vi "TestStandSoftware.vi"(11 "notifier":refnum<notifier>) -> ()   [LabVIEW 2025]
doc: "This is the main VI for the configuration editor.Copyright 2017 National Instruments Corporation\n\nLicensed under the Apache License, Version 2.0 (the \"License\"); you may not use this file except in compliance with the License. You may obtain a copy of the License at http://www.apache.org/licenses/LICENSE-2.0\nUnless required by applicable law or agreed to in writing, software distributed under the License is distributed on an \"AS IS\" BASIS, WITHOUT WARRANTIES OR CONDITIONS OF ANY KIND, either express or implied. See the License for the specific language governing permissions and limitations under the License."
uses:
  Configuration Tools/Controls/StateCluster.ctl
  Users/Public/Documents/Sandia National Labs/TSS Plugin/CEF.lvlibp/Repository/CEF_Repository.lvclass
  Users/Public/Documents/Sandia National Labs/TSS Plugin/CEF.lvlibp/Node/NodeRef.ctl
  Users/Public/Documents/Sandia National Labs/TSS Plugin/CEF.lvlibp/Node/CEF_Node.lvclass
  Users/Public/Documents/Sandia National Labs/TSS Plugin/CEF.lvlibp/Node/StandardEvents.ctl
  Configuration Tools/Controls/FilePaths.ctl
  Users/Public/Documents/Sandia National Labs/TSS Plugin/CEF.lvlibp/glyph manager/glyph manager.ctl
  <vilib>/Utility/config.llb/Config Data RefNum.ctl
  Configuration Tools/Controls/AddMessage.ctl
  Configuration Tools/Controls/MoveMessage.ctl
  Users/Public/Documents/Sandia National Labs/TSS Plugin/CEF.lvlibp/hierarchy repo/CEF_HierarchyRepo.lvclass
  C:/Users/Public/Documents/Sandia National Labs/TSS Plugin/CEF.lvlibp/Repository/CEF_Repository.lvclass
  Users/Public/Documents/Sandia National Labs/TSS Plugin/System.lvlibp/System/System.lvclass
  Users/Public/Documents/Sandia National Labs/TSS Plugin/CEF.lvlibp/serializable node/CEF_serializable node.lvclass
  C:/Users/Public/Documents/Sandia National Labs/TSS Plugin/CEF.lvlibp/Node/CEF_Node.lvclass
  <vilib>/National Instruments/Asynchronous TDMS Logger/_Typedefs/Multiple Files Configuration.ctl
  <vilib>/National Instruments/Asynchronous TDMS Logger/_Typedefs/Multiple Files Action.ctl
  <vilib>/National Instruments/Asynchronous TDMS Logger/_Typedefs/Old Files Configuration.ctl
  <vilib>/National Instruments/Asynchronous TDMS Logger/_Typedefs/Folder Size Limit Reached.ctl
  ce7dbd15-68e1-444f-b0a0-607e461cde1a.vi
  Control Globals.vi
  Users/Public/Documents/Sandia National Labs/TSS Plugin/CEF.lvlibp/Node/ReadChildren.vi
  Users/Public/Documents/Sandia National Labs/TSS Plugin/CEF.lvlibp/Node/ReadNodeClass.vi
  C:/Users/Public/Documents/Sandia National Labs/TSS Plugin/CEF.lvlibp/hierarchy repo/CEF_HierarchyRepo.lvclass
  C:/Users/Public/Documents/Sandia National Labs/TSS Plugin/CEF.lvlibp/serializable node/CEF_serializable node.lvclass
  Configuration Tools/Config Tool.lvlib
  Users/Public/Documents/Sandia National Labs/TSS Plugin/CEF.lvlibp
  <vilib>/Utility/config.llb/NI_LVConfig.lvlib
  <vilib>/National Instruments/Asynchronous TDMS Logger/TDMS Logger.lvclass
panel:
  in  "Record":bool
  out "Time":dbl format="%<%H:%M:%S>t"
  in  "Initialize Engines":bool
  in  "File Menu":bool
  in  "TreeView":string(tree)="NID741343233"
  in  "ExecutionView Manager":refnum<k7>(container)
  in  "SequenceFileView Manager":refnum<k7>(container)
  in  "Application Manager":refnum<k7>(container)
  in  "Close Executions Btn":refnum<k7>(container)
  in  "Close Sequence File Btn":refnum<k7>(container)
  in  "Open Sequence File Btn":refnum<k7>(container)
  in  "Run Selected Sequence Btn":refnum<k7>(container)
  in  "Entry Point 2 Btn":refnum<k7>(container)
  in  "Entry Point 1 Btn":refnum<k7>(container)
  in  "Executions ComboBox":refnum<k7>(container) caption="Executions"
  in  "Sequences ComboBox":refnum<k7>(container) caption="Sequences"
  in  "Sequence Files ComboBox":refnum<k7>(container) caption="Sequence Files"
  in  "Execution View":refnum<k7>(container)
  in  "Terminate All Btn":refnum<k7>(container)
  in  "Break/Resume Btn":refnum<k7>(container)
  in  "Terminate/Restart Btn":refnum<k7>(container)
  in  "Report Viewer":refnum<k7>(container)
  in  "TS Pane":bool
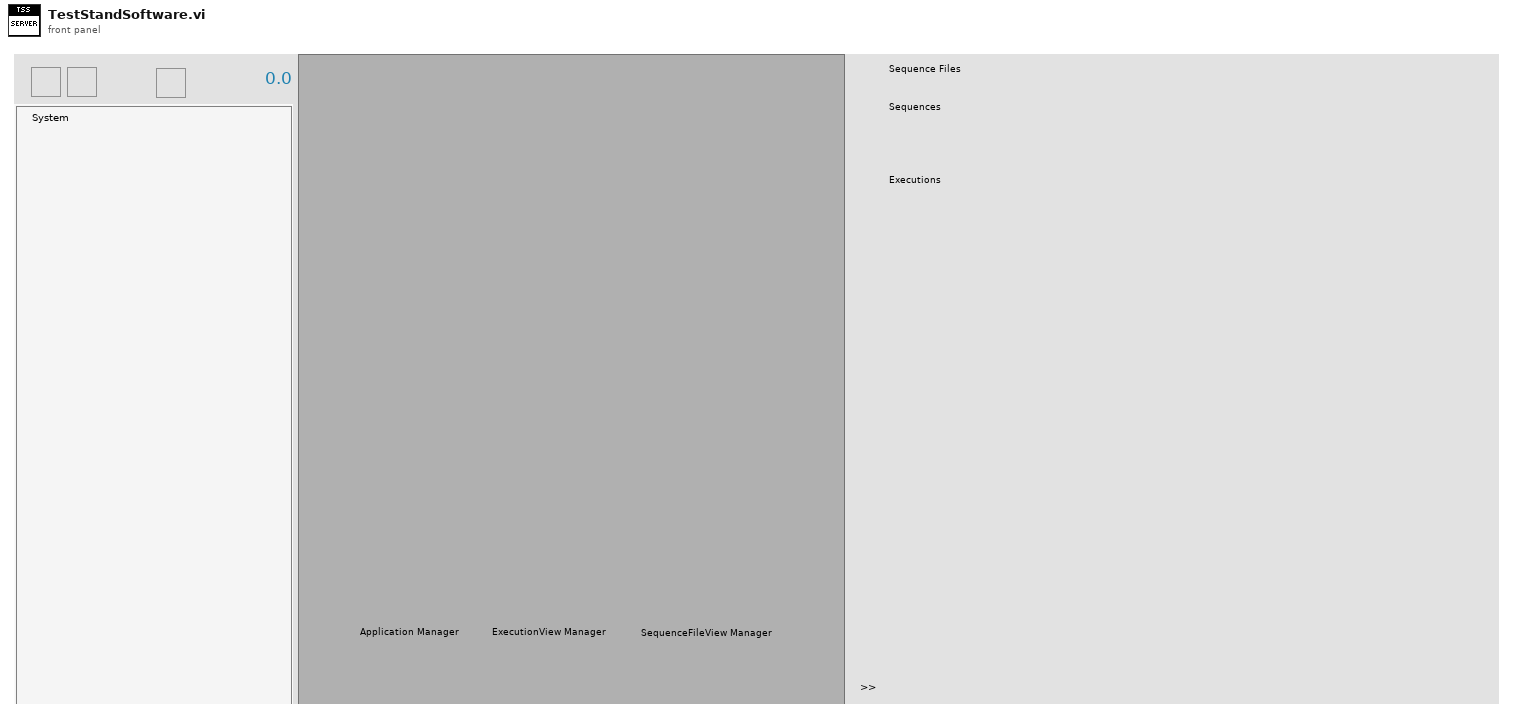
[diagram p1: front panel]
types:
  T1 = typedef "Config Tool.lvlib/StateCluster.ctl" = cluster{"repository":refnum<class "CEF_Repository.lvclass">, "root":T2, "standard events":T3, "paths":T4, "glyph manager":T5, "current path":path, "unsaved changes":bool, "menu":refnum<k9>, "Error Log":refnum<file>, "INI file ref":T6, "Record":bool, "tdms file":refnum<k34>}
  T2 = typedef "CEF.lvlibp/CEF_Node.lvclass/NodeRef.ctl" = refnum<data-value>
  T3 = typedef "CEF.lvlibp/CEF_Node.lvclass/StandardEvents.ctl" = cluster{"user event":refnum<user-event>, "node change":refnum<user-event>, "cache state":refnum<user-event>, "refresh UI":refnum<user-event>, "stop event":refnum<user-event>, "Quit App":refnum<user-event>}
  T4 = typedef "Config Tool.lvlib/FilePaths.ctl" = cluster{"Configuration":path, "Plugin":path, "Glyphs":path, "Data":path, "Error Log":path}
  T5 = typedef "CEF.lvlibp/glyph manager.ctl" = cluster{"search paths":path[], "glyph map":variant, "base glyphs":cluster{"image type":i32, "image depth":i32, "image":u8[], "mask":u8[], "colors":u32[], "Rectangle":cluster{"left":i16, "top":i16, "right":i16, "bottom":i16}}[], "desired overlays":string[]}
  T6 = typedef "NI_LVConfig.lvlib/Config Data RefNum.ctl" = refnum<k1>
  T7 = cluster{"user event":refnum<user-event>, "node change":refnum<user-event>, "cache state":refnum<user-event>, "refresh UI":refnum<user-event>, "stop event":refnum<user-event>, "Quit App":refnum<user-event>}
  T8 = typedef "Config Tool.lvlib/AddMessage.ctl" = cluster{"subNode":string, "Node ID":string}
  T9 = typedef "Config Tool.lvlib/MoveMessage.ctl" = cluster{"node ref":T2, "new parent":T2, "Index":i32}
  T10 = typedef "TDMS Logger.lvlib/TDMS Logger.lvclass/Old Files Configuration.ctl" = cluster{"Action on Max Folder Size":T11, "Max # Files in Folder":i32}
  T11 = typedef "TDMS Logger.lvlib/TDMS Logger.lvclass/Folder Size Limit Reached.ctl" = enum16{"Do Nothing", "Remove Oldest Files"}
  T12 = typedef "TDMS Logger.lvlib/TDMS Logger.lvclass/Multiple Files Configuration.ctl" = cluster{"Multiple Files Action":T13, "Max File Size (MB)":dbl, "Max Time in File (s)":dbl}
  T13 = typedef "TDMS Logger.lvlib/TDMS Logger.lvclass/Multiple Files Action.ctl" = enum16{"Seperate based on size", "Seperate based on time", "Single file"}
  T14 = cluster{"Message Name":string, "data string":string}
  T15 = typedef "LVPoint32TypeDef.ctl" = cluster{"Horizontal":i32, "Vertical":i32}
  T16 = cluster{"data name":string, "drag data":variant}[]
  T17 = cluster{"removable":bool, "movable":bool, "duplicate":bool}
  T18 = cluster{"message name":string, "data string":string}
  T19 = enum16{"Start Timer", "Read Time", "Pause", "Resume"}
  T20 = enum16{"open", "open or create", "create or replace", "create", "open (read-only)"}
  T21 = cluster{"search paths":path[], "glyph map":variant, "base glyphs":cluster{"image type":i32, "image depth":i32, "image":u8[], "mask":u8[], "colors":u32[], "Rectangle":cluster{"left":i16, "top":i16, "right":i16, "bottom":i16}}[], "desired overlays":string[]}
  T22 = cluster{"ID":string, "parent ID":string, "node type":string, "text":string, "additional text":string, "glyph":string, "depth":i32, "glyph overlay":string}[]
  T23 = cluster{"ID":string, "parent ID":string, "node type":string, "text":string, "additional text":string, "glyph":string, "depth":i32, "glyph overlay":string}
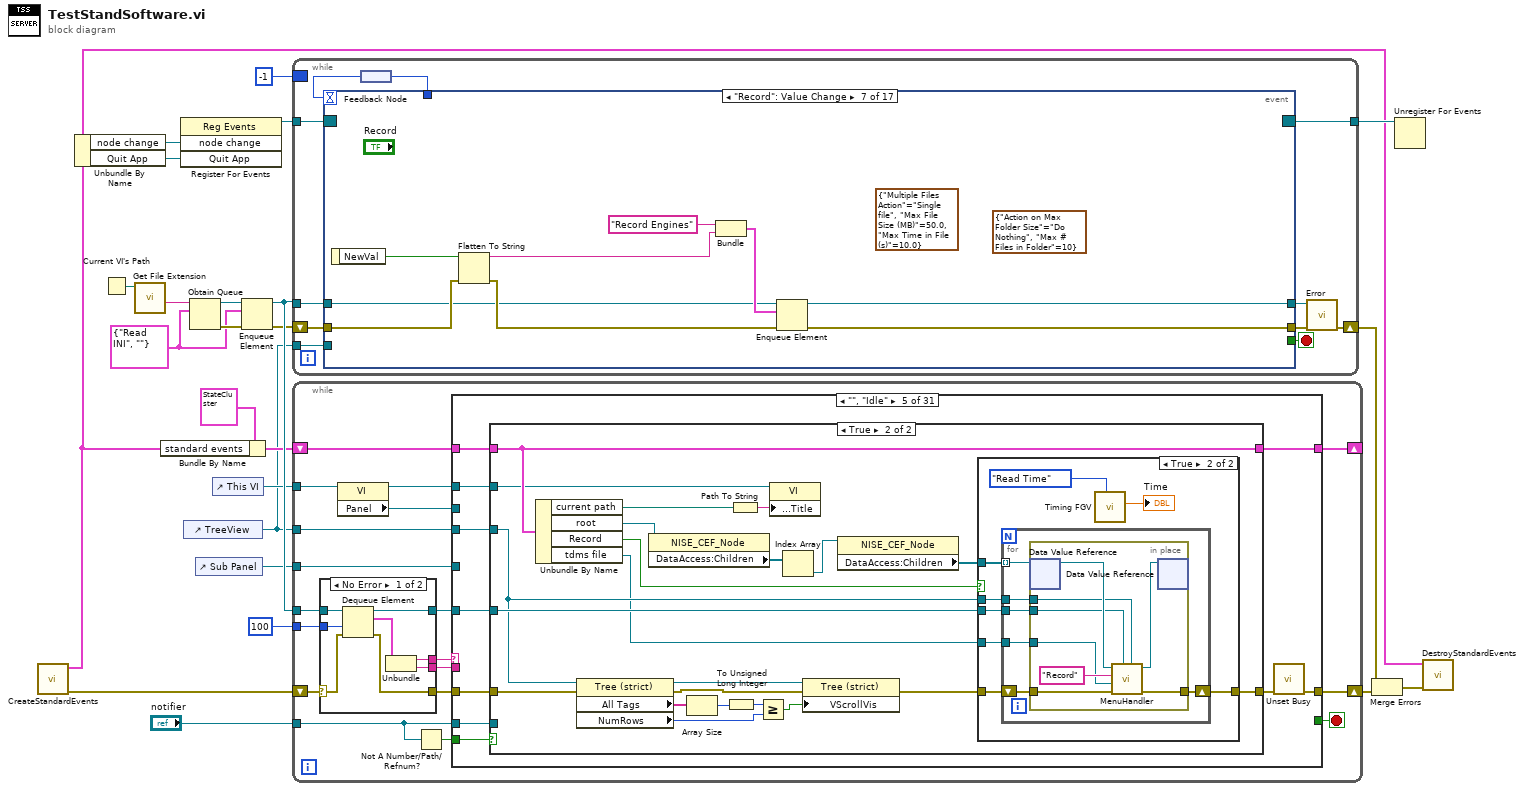
[diagram p0: block diagram]
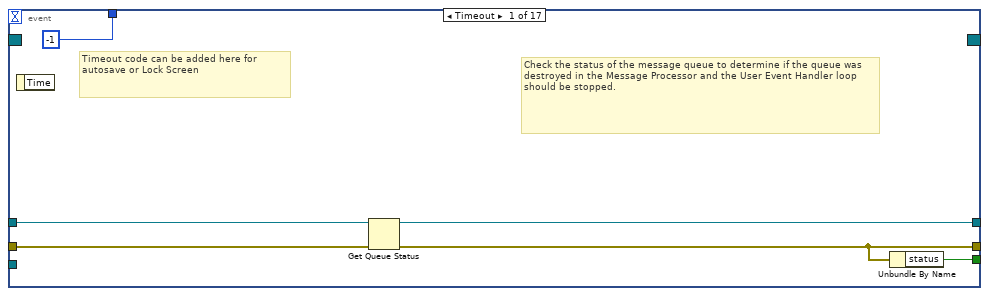
[diagram p2: hidden frame]
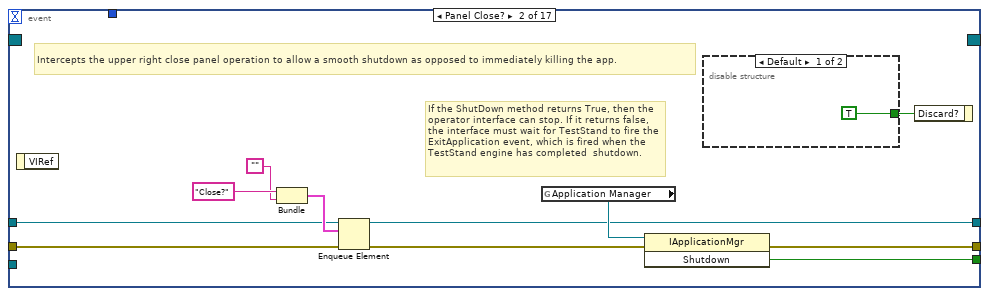
[diagram p3: hidden frame]
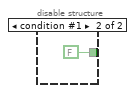
[diagram p4: hidden frame]
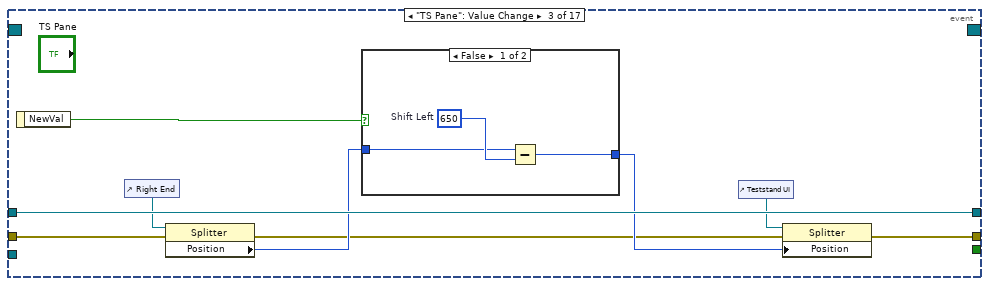
[diagram p5: hidden frame]
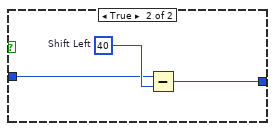
[diagram p6: hidden frame]
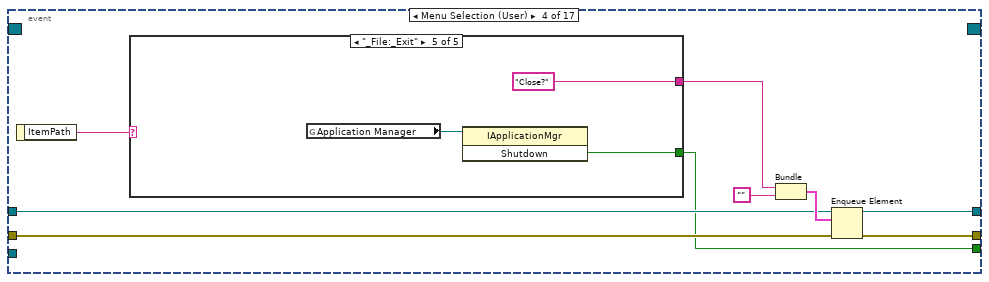
[diagram p7: hidden frame]
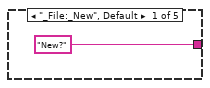
[diagram p8: hidden frame]
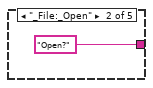
[diagram p9: hidden frame]
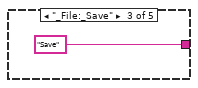
[diagram p10: hidden frame]
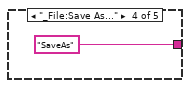
[diagram p11: hidden frame]
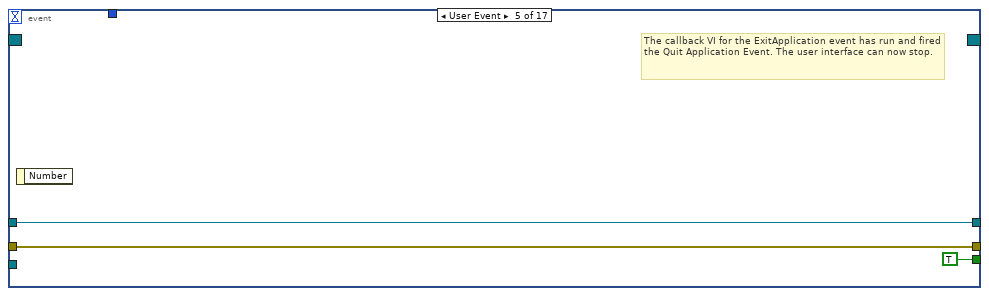
[diagram p12: hidden frame]
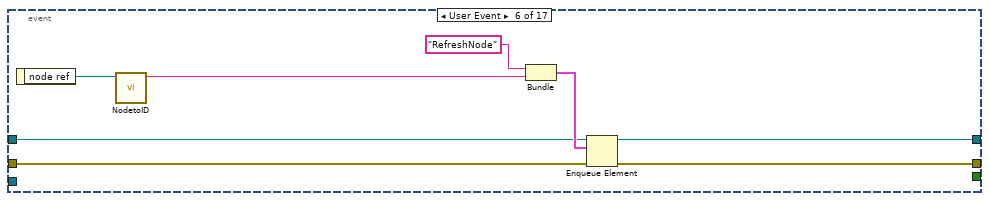
[diagram p13: hidden frame]
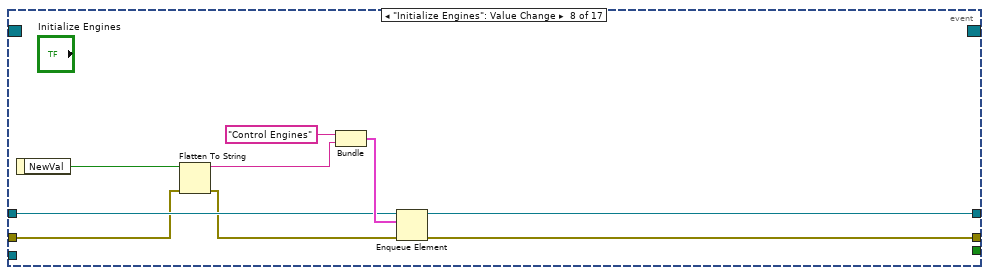
[diagram p14: hidden frame]
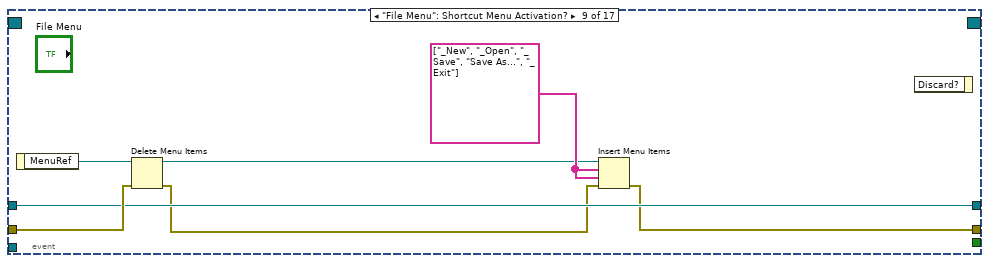
[diagram p15: hidden frame]
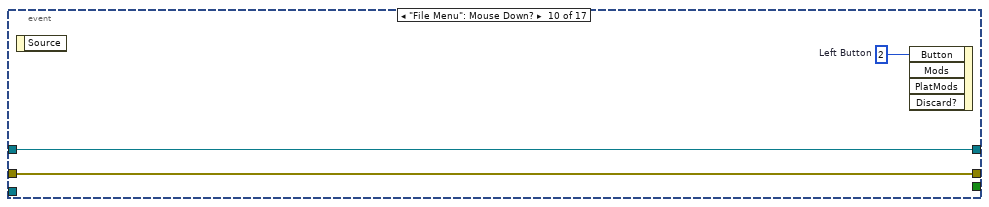
[diagram p16: hidden frame]
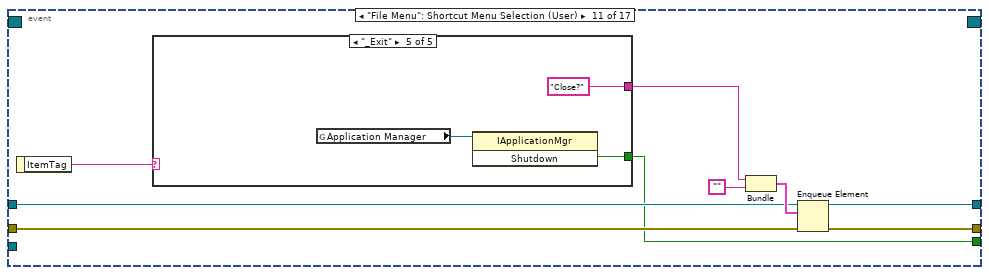
[diagram p17: hidden frame]
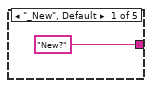
[diagram p18: hidden frame]
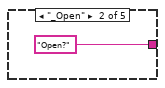
[diagram p19: hidden frame]
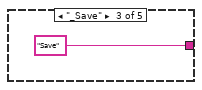
[diagram p20: hidden frame]
diagram:
  w10 = cluster{"message":string, "string":string} {"message"="Read INI", "string"=""}
  n1 = call "CreateStandardEvents.vi"() -> ("error out"=w14:errorcluster, "standard events"=w16:T7)  [unwired: 10 in]
  n2 = Unbundle By Name(w16) -> ("node change"=w15:refnum<user-event>, "Quit App"=w1:refnum<user-event>)
  n3 = Current VI's Path() -> (path=w21:path)
  n4 = call <vilib>:"Get File Extension.vi"("file"=w21) -> ("filename without extension"=w11:string)  [unwired: 6 in, 4 out]
  n5 = Bundle By Name(cluster=T1 {"repository"=refnum, "root"=refnum, "standard events"={"user event"=refnum, "node change"=refnum, "cache state"=refnum, "refresh UI"=refnum, "stop event"=refnum, "Quit App"=refnum}, "paths"={"Configuration"=path "", "Plugin"=path "", "Glyphs"=path "", "Data"=path "", "Error Log"=path ""}, "glyph manager"={"search paths"=[], "glyph map"=variant, "base glyphs"=[], "desired overlays"=[]}, "current path"=path "", "unsaved changes"=FALSE, "menu"=refnum, "Error Log"=refnum, "INI file ref"=refnum, "Record"=FALSE, "tdms file"=refnum} ("state cluster"), "standard events"=w16) -> (w4:T1)
  n6 = register-events(w15, w1) -> (reference out=w2:refnum<event-registration>)  [unwired: 2 in, 1 out]
  n7 = control-ref of="TreeView"() -> (w3:refnum<vi>)
  n8 = Obtain Queue(name (unnamed)=w11, element data type=w10) -> (queue out=w12:refnum<queue>, error out=w13:errorcluster)  [unwired: 3 in, 1 out]
  n9 = control-ref of="Sub Panel"() -> (w5:refnum<vi>)
  n10 = control-ref of="This VI"() -> (w6:refnum<vi>)
  n11 = Enqueue Element(queue=w12, element=w10, error in (no error)=w13) -> (queue out=w9:refnum<queue>, error out=w8:errorcluster)  [unwired: 1 in, 1 out]
  n12 = while "User Interface Event Handler" {
    tunnel: w9 -> [w34]
    tunnel: w3 -> [w29]
    tunnel: w2 -> [w28]
    tunnel: [w27] -> w17
    border: -1 -> [_]
    shift-right: [w31] -> w22
    shift-left: w8 -> [w35]
    stop <- w33 stop-if-true
    n13 = feedback #1() -> (w25:i32)
    n14 = event shown="[6] \"Record\": Value Change" {
      selector: w28 -> [_ _ _ _ _ _ _ _ _ _ _ _ _ _ _ _ _]
      dyn-events: [_ _ _ _ _ _ _ _ _ _ _ _ _ _ _ _ _] -> w27
      timeout: w25 -> [_ _ _ _ _ _ _ _ _ _ _ _ _ _ _ _ _]
      tunnel: [w36 w49 _ w71 TRUE ("Shutdown") _ _ _ _ _ w127 _ _ _ _ _ _] -> w33
      tunnel: [w37 w51 w62 w78 w90 w97 w101 w108 w117 w124 w128 w159 w182 w211 w239 w250 w286] -> w32
      tunnel: w35 -> [w38 w45 w57 w72 w90 w91 w103 w110 w123 w124 w129 w150 w181 w210 w237 w251 w287]
      tunnel: w34 -> [w41 w44 w64 w73 w89 w93 w102 w114 w121 w125 w131 w148 w177 w209 w236 w245 w280]
      tunnel: [w40 w43 w64 w77 w89 w92 w100 w113 w121 w125 w130 w148 w176 w209 w236 _ w279] -> w30
      tunnel: w29 -> [_ _ _ _ _ _ _ _ _ _ _ w146 _ _ _ _ _]
      tunnel: [-1 _ _ _ _ _ _ _ _ _ _ _ _ _ _ _ _] -> w26
      event Timeout {
        # "Check the status of the message queue to determine if the queue was destroyed in the Message Processor and the User Event Handler loop should be stopped."
        # "Timeout code can be added here for autosave or Lock Screen"
        n15 = event-data() -> ()  [unwired: 1 in, 1 out]
        n16 = Get Queue Status(queue=w41, error in (no error)=w38) -> (queue out=w40:refnum<queue>, error out=w37:errorcluster)  [unwired: 1 in, 6 out]
        n17 = Unbundle By Name(w37) -> ("status"=w36:bool)
      }
      event Panel Close? {
        # "If the ShutDown method returns True, then the operator interface can stop. If it returns false, the interface must wait for TestStand to fire the ExitApplication event, which is fired when the TestStand engine has completed  shutdown."
        # "Intercepts the upper right close panel operation to allow a smooth shutdown as opposed to immediately killing the app."
        n18 = event-data() -> ()  [unwired: 1 in, 1 out]
        n19 = Bundle("Close?", "") -> (w48:cluster{string, string})  [unwired: 1 in]
        n20 = Enqueue Element(queue=w44, element=w48, error in (no error)=w45) -> (queue out=w43:refnum<queue>, error out=w42:errorcluster)  [unwired: 1 in, 1 out]
        n21 = global read "Control Globals.vi" "Application Manager"() -> (w50:refnum<k7>)
        n22 = global read "Control Globals.vi" "Application Manager"() -> (w52:refnum<k7>)
        n23 = invoke class="IApplicationMgr" method="Shutdown"(reference=w50, error in=w42) -> ()  [unwired: 1 in, 3 out]
        n24 = invoke class="IApplicationMgr" method="Shutdown"(reference=w52) -> (error out=w51:errorcluster, "Shutdown"=w49:bool)  [unwired: 2 in, 1 out]
        n25 = disable-structure shown="Default" {
          disable-tunnel: [TRUE FALSE] -> w53
          frame condition #0 (active) {
          }
          frame condition #1 {
          }
        }
        n26 = event-data("Discard?"=w53) -> ()  [unwired: 1 in, 1 out]
      }
      event "TS Pane": Value Change {
        n27 = event-data() -> ("NewVal"=w60:bool)  [unwired: 1 in]
        n28 = control-ref of="Right End"() -> (w61:refnum<vi>)
        n29 = property class="Splitter"(reference=w61, error in=w57) -> (error out=w56:errorcluster, "Position"=w59:i32)  [unwired: 1 out]
        n30 = case shown="False" w60 {
          tunnel: w59 -> [w66 w69]
          tunnel: [w65 w68] -> w58
          frame False {
            w67 = 650  # Shift Left
            n31 = Subtract(x=w66, y=w67) -> (x-y=w65:i32)
          }
          frame True {
            w70 = 40  # Shift Left
            n32 = Subtract(x=w69, y=w70) -> (x-y=w68:i32)
          }
        }
        n33 = control-ref of="Teststand UI"() -> (w63:refnum<vi>)
        n34 = property class="Splitter"(reference=w63, error in=w56, "Position"=w58) -> (error out=w62:errorcluster)  [unwired: 1 out]
      }
      event Menu Selection (User) {
        n35 = event-data() -> ("ItemPath"=w79:string)  [unwired: 1 in]
        n36 = case shown="\"_File:_Exit\"" w79 {
          tunnel: ["New?" ("Message Name") "Open?" ("Message Name") "Save" ("Message Name") "SaveAs" ("Message Name") "Close?" ("Message Name")] -> w75
          tunnel: [_ _ _ _ w84] -> w71
          frame "_File:_New", Default {
          }
          frame "_File:_Open" {
          }
          frame "_File:_Save" {
          }
          frame "_File:Save As..." {
          }
          frame "_File:_Exit" {
            n37 = global read "Control Globals.vi" "Application Manager"() -> (w85:refnum<k7>)
            n38 = global read "Control Globals.vi" "Application Manager"() -> (w86:refnum<k7>)
            n39 = invoke class="IApplicationMgr" method="Shutdown"(reference=w85) -> ("Shutdown"=w84:bool)  [unwired: 2 in, 2 out]
            n40 = invoke class="IApplicationMgr" method="Shutdown"(reference=w86) -> ()  [unwired: 2 in, 3 out]
          }
        }
        n41 = Bundle("Message Name"=w75, "") -> (w74:cluster{"Message Name":string, string})  [unwired: 1 in]
        n42 = Enqueue Element(queue=w73, element=w74, error in (no error)=w72) -> (queue out=w77:refnum<queue>, error out=w78:errorcluster)  [unwired: 1 in, 1 out]
      }
      event User Event {
        # "The callback VI for the ExitApplication event has run and fired the Quit Application Event. The user interface can now stop."
        n43 = event-data() -> ()  [unwired: 1 in, 1 out]
      }
      event User Event {
        n44 = event-data() -> ("node ref"=w98:refnum<data-value>)  [unwired: 1 in]
        n45 = call "NodetoID.vi"("node ref"=w98) -> ("ID"=w94:string)  [unwired: 9 in, 1 out]
        n46 = Bundle("message name"="RefreshNode", "ID"=w94) -> (w95:cluster{"message name":string, "ID":string})  [unwired: 1 in]
        n47 = Enqueue Element(queue=w93, element=w95, error in (no error)=w91) -> (queue out=w92:refnum<queue>, error out=w97:errorcluster)  [unwired: 1 in, 1 out]
      }
      event "Record": Value Change {
        (unwired) T10 {"Action on Max Folder Size"=enum."Do Nothing", "Max # Files in Folder"=10} ("Old Files Configuration")
        (unwired) T12 {"Multiple Files Action"=enum."Single file", "Max File Size (MB)"=50.0, "Max Time in File (s)"=10.0} ("Multiple Files Configuration")
        n48 = event-data() -> ("NewVal"=w99:bool)  [unwired: 1 in]
        n49 = Flatten To String(anything=w99, error in (no error)=w103) -> (data string=w105:string, error out=w104:errorcluster)  [unwired: 2 in, 1 out]
        n50 = Bundle("Message Name"="Record Engines", "data string"=w105) -> (w107:T14)  [unwired: 1 in]
        n51 = Enqueue Element(queue=w102, element=w107, error in (no error)=w104) -> (queue out=w100:refnum<queue>, error out=w101:errorcluster)  [unwired: 1 in, 1 out]
      }
      event "Initialize Engines": Value Change {
        n52 = event-data() -> ("NewVal"=w112:bool)  [unwired: 1 in]
        n53 = Flatten To String(anything=w112, error in (no error)=w110) -> (data string=w111:string, error out=w109:errorcluster)  [unwired: 2 in, 1 out]
        n54 = Bundle("Message Name"="Control Engines", "data string"=w111) -> (w116:T14)  [unwired: 1 in]
        n55 = Enqueue Element(queue=w114, element=w116, error in (no error)=w109) -> (queue out=w113:refnum<queue>, error out=w108:errorcluster)  [unwired: 1 in, 1 out]
      }
      event "File Menu": Shortcut Menu Activation? {
        w120 = string[] ["_New", "_Open", "_Save", "Save As...", "_Exit"] ("item names")
        n56 = event-data() -> ("MenuRef"=w122:refnum<k9>)  [unwired: 1 in]
        n57 = Delete Menu Items(6:w123, 9:w122) -> (0:w118:errorcluster, 3:w119:refnum<k9>)  [unwired: 2 in]
        n58 = Insert Menu Items(6:w118, 7:w120, 8:w120, 9:w119) -> (0:w117:errorcluster)  [unwired: 2 in, 2 out]
        n59 = event-data() -> ()  [unwired: 2 in, 1 out]
      }
      event "File Menu": Mouse Down? {
        w126 = u16 2  # Left Button
        n60 = event-data() -> ()  [unwired: 1 in, 1 out]
        n61 = event-data("Button"=w126) -> ()  [unwired: 4 in, 1 out]
      }
      event "File Menu": Shortcut Menu Selection (User) {
        n62 = event-data() -> ("ItemTag"=w135:string)  [unwired: 1 in]
        n63 = case shown="\"_Exit\"" w135 {
          tunnel: ["New?" ("Message Name") "Open?" ("Message Name") "Save" ("Message Name") "SaveAs" ("Message Name") "Close?" ("Message Name")] -> w133
          tunnel: [_ _ _ _ w141] -> w127
          frame "_New", Default {
          }
          frame "_Open" {
          }
          frame "_Save" {
          }
          frame "Save As..." {
          }
          frame "_Exit" {
            n64 = global read "Control Globals.vi" "Application Manager"() -> (w142:refnum<k7>)
            n65 = global read "Control Globals.vi" "Application Manager"() -> (w143:refnum<k7>)
            n66 = invoke class="IApplicationMgr" method="Shutdown"(reference=w142) -> ("Shutdown"=w141:bool)  [unwired: 2 in, 2 out]
            n67 = invoke class="IApplicationMgr" method="Shutdown"(reference=w143) -> ()  [unwired: 2 in, 3 out]
          }
        }
        n68 = Bundle("Message Name"=w133, "") -> (w132:cluster{"Message Name":string, string})  [unwired: 1 in]
        n69 = Enqueue Element(queue=w131, element=w132, error in (no error)=w129) -> (queue out=w130:refnum<queue>, error out=w128:errorcluster)  [unwired: 1 in, 1 out]
      }
      event "TreeView": Shortcut Menu Activation? {
        n70 = event-data() -> ("MenuRef"=w149:refnum<k9>, "CtlRef"=w162:refnum<vi>, "Coords"=w161:T15)  [unwired: 1 in]
        n71 = invoke class="Tree (strict)" method="Point To Row Column"(reference=w162, "Point"=w161) -> ("Tag"=w160:string)  [unwired: 6 in, 7 out]
        n72 = property class="Tree (strict)"(reference=w146, error in=w150) -> (error out=w147:errorcluster, "Allow Editing Cells"=w145:bool)  [unwired: 1 out]
        n73 = call "IDtoNode.vi"("error in"=w147, "ID"=w160) -> ("error out"=w155:errorcluster, "invalid Id"=w153:bool, "node ref"=w158:refnum<data-value>)  [unwired: 7 in]
        n74 = Not(x=w153) -> (.not. x?=w144:bool)
        n75 = And(x=w144, y=w145) -> (x .and. y?=w152:bool)
        n76 = case shown="False" w152 {
          tunnel: w158 -> [_ w170]
          tunnel: w149 -> [_ w169]
          tunnel: [_ w168] -> w157
          tunnel: [_ w167] -> w156
          tunnel: w155 -> [w164 w166]
          tunnel: [w164 w166] -> w154
          tunnel: [TRUE ("Discard?") FALSE ("Discard?")] -> w151
          frame False {
          }
          frame True {
            n77 = in-place {
              in-place-border: w169 -> [w173]
              in-place-border: [w171] -> w168
              n78 = in-place-dvr #2(w170) -> (w175:refnum<class "CEF_Node.lvclass">, w172:errorcluster)
              n79 = call-dynamic "ShortcutMenu.vi"("error in"=w172, "menu ref in"=w173, "CEF_Node in"=w175) -> ("error out"=w171:errorcluster, "CEF_Node out"=w174:refnum<class "CEF_Node.lvclass">)  [unwired: 6 in, 1 out]
              n80 = in-place-dvr #2(w174) -> (w167:errorcluster)  [unwired: 1 out]
            }
          }
        }
        n81 = Merge Errors(w156, w157, w154) -> (w159:errorcluster)
        n82 = event-data("Discard?"=w151) -> ()  [unwired: 1 in, 1 out]
      }
      event "TreeView": Shortcut Menu Selection (User) {
        n83 = event-data() -> ("ItemPath"=w184:string, "CtlRef"=w187:refnum<vi>, "Coords"=w188:T15)  [unwired: 1 in]
        n84 = invoke class="Tree (strict)" method="Point To Row Column"(reference=w187, "Point"=w188) -> ("Tag"=w183:string)  [unwired: 6 in, 7 out]
        n85 = Match Pattern(string=w184, regular expression=":") -> (before substring=w186:string, after substring=w185:string)  [unwired: 1 in, 2 out]
        n86 = case shown="Default" w186 {
          selector: w186 -> [w192 _ _ _ _ _]
          tunnel: w185 -> [_ _ _ w202 _ _]
          tunnel: w183 -> [w193 w195 w197 w203 w205 w208]
          tunnel: ["CustomMenuAction" ("Message Name") "RemoveNode" ("Message Name") "Duplicate" ("Message Name") "AddNode" ("Message Name") "Import Engine" ("Message Name") "Export Engine" ("Message Name")] -> w179
          tunnel: [w190 w195 w197 w199 w205 w208] -> w180
          frame Default {
            # "Right click menu"
            n87 = Concatenate Strings(w192, ":" ("string"), w193) -> (w190:string)
          }
          frame "Remove" {
          }
          frame "Duplicate" {
          }
          frame "Add" {
            n88 = Bundle By Name(cluster=T8 {"subNode"="", "Node ID"=""} ("input cluster"), "subNode"=w202, "Node ID"=w203) -> (w200:T8)
            n89 = Flatten To String(anything=w200) -> (data string=w199:string)  [unwired: 3 in, 2 out]
          }
          frame "Import" {
          }
          frame "Export" {
          }
        }
        n90 = Bundle("Message Name"=w179, "Tag"=w180) -> (w178:cluster{"Message Name":string, "Tag":string})  [unwired: 1 in]
        n91 = Enqueue Element(queue=w177, element=w178, error in (no error)=w181) -> (queue out=w176:refnum<queue>, error out=w182:errorcluster)  [unwired: 1 in, 1 out]
      }
      event "TreeView": Drag Starting? {
        n92 = event-data() -> ("Data"=w218:T16, "CtlRef"=w220:refnum<vi>, "Coords"=w219:T15)  [unwired: 1 in]
        n93 = invoke class="Tree (strict)" method="Point To Row Column"(reference=w220, "Point"=w219) -> ("Tag"=w217:string)  [unwired: 6 in, 7 out]
        n94 = call "IDtoNode.vi"("error in"=w210, "ID"=w217) -> ("error out"=w212:errorcluster, "invalid Id"=w216:bool, "node ref"=w215:refnum<data-value>)  [unwired: 7 in]
        n95 = case shown="True" w216 {
          tunnel: w215 -> [w228 _]
          tunnel: [w225 TRUE ("Removable")] -> w213
          tunnel: w212 -> [w224 w234]
          tunnel: [w221 w234] -> w211
          frame False {
            n96 = in-place {
              in-place-border: [w231] -> w227
              in-place-border: w224 -> [w230]
              in-place-border: [w229] -> w223
              n97 = in-place-dvr #3(w228) -> (w233:refnum<class "CEF_Node.lvclass">)  [unwired: 1 out]
              n98 = call-dynamic "EditOptions.vi"("error in"=w230, "CEF_Node in"=w233) -> ("error out"=w229:errorcluster, "edit options"=w231:T17, "CEF_Node out"=w232:refnum<class "CEF_Node.lvclass">)  [unwired: 6 in, 1 out]
              n99 = in-place-dvr #3(w232) -> (w222:errorcluster)  [unwired: 1 out]
            }
            n100 = Unbundle By Name(w227) -> ("movable"=w226:bool)
            n101 = Merge Errors(w222, w223) -> (w221:errorcluster)
            n102 = Not(x=w226) -> (.not. x?=w225:bool)
          }
          frame True {
          }
        }
        n103 = event-data("Data"=w218, "Drag Mode"=enum32{"copy or move", "copy only", "move only"}."move only", "Discard?"=w213) -> ()  [unwired: 1 in, 1 out]
      }
      event "TreeView": event type 3.0.xa000003a {
        n104 = event-data() -> ("CtlRef"=w244:refnum<vi>, "Coords"=w241:T15)  [unwired: 1 in]
        n105 = invoke class="Tree (strict)" method="Point To Row Column"(reference=w244, "Point"=w241) -> (reference out=w243:refnum<vi>, "Tag"=w242:string)  [unwired: 6 in, 6 out]
        n106 = call "ValidDragDrop.vi"("error in"=w237, "Reorder"=TRUE, "drag over"=w242, "Tree Ref in"=w243) -> ("Error Out"=w239:errorcluster, "Accepted"=w240:bool)  [unwired: 6 out]
        n107 = event-data("Accepted?"=w240) -> ()  [unwired: 1 in, 1 out]
      }
      event "TreeView": Drop {
        n108 = event-data() -> ("CtlRef"=w262:refnum<vi>, "Coords"=w261:T15)  [unwired: 1 in]
        n109 = invoke class="Tree (strict)" method="Point To Row Column"(reference=w262, "Point"=w261) -> (reference out=w260:refnum<vi>, "Tag"=w257:string)  [unwired: 6 in, 6 out]
        n110 = call "ValidDragDrop.vi"("error in"=w251, "Reorder"=TRUE, "drag over"=w257, "Tree Ref in"=w260) -> ("Error Out"=w249:errorcluster, "Accepted"=w255:bool, "Drag"=w259:string, "Tree Ref out"=w264:refnum<vi>, "Moved Node"=w253:refnum<data-value>, "Position"=w252:i32, "Parent Node"=w254:refnum<data-value>, "Parent"=w256:string)
        n111 = case shown="True" w255 {
          tunnel: w259 -> [_ w276]
          tunnel: w264 -> [_ w278]
          tunnel: [_ TRUE] -> w263
          tunnel: w256 -> [_ w275]
          tunnel: w253 -> [_ w274]
          tunnel: w254 -> [_ w273]
          tunnel: w252 -> [_ w272]
          tunnel: ["Idle" ("message name") "Move" ("message name")] -> w248
          tunnel: [_ w267] -> w247
          frame False {
          }
          frame True {
            n112 = invoke class="Tree (strict)" method="Edit Tree Items.Move Item"(reference=w278, "tag"=w276, "New Parent"=w275, "New Position"=0, "Carry Children"=FALSE ("Carry Children?")) -> ()  [unwired: 2 in, 7 out]
            n113 = Bundle By Name(cluster=T9 {"node ref"=refnum, "new parent"=refnum, "Index"=0}, "Index"=w272, "node ref"=w274, "new parent"=w273) -> (w269:T9)
            n114 = Flatten To String(anything=w269) -> (data string=w267:string)  [unwired: 3 in, 2 out]
          }
        }
        n115 = Bundle("message name"=w248, "data string"=w247) -> (w246:T18)  [unwired: 1 in]
        n116 = event-data("Accepted?"=w263) -> ()  [unwired: 1 in, 1 out]
        n117 = Enqueue Element(queue=w245, element=w246, error in (no error)=w249) -> (error out=w250:errorcluster)  [unwired: 1 in, 2 out]
      }
      event "TreeView": Value Change {
        # "Don't remove"
        n118 = event-data() -> ("NewVal"=w282:string)  [unwired: 1 in]
        n119 = call "Stall Data Flow.vim"("value in"=w287, "milliseconds to wait"=u32 100) -> ("value out"=w285:errorcluster)  [unwired: 1 out]
        n120 = Bundle("Message Name"="ActivateNode", "NewVal"=w282) -> (w281:cluster{"Message Name":string, "NewVal":string})  [unwired: 1 in]
        n121 = Enqueue Element(queue=w280, element=w281, error in (no error)=w285) -> (queue out=w279:refnum<queue>, error out=w286:errorcluster)  [unwired: 1 in, 1 out]
      }
    }
    n122 = feedback-in #1(w26) -> ()
    n123 = call "Error.vi"("error in (no error)"=w32, "main queue"=w30) -> ("error out"=w31:errorcluster)  [unwired: 9 in]
  }
  n124 = while "Message Processor" {
    shift-right: [w304] -> _
    shift-left: w4 -> [w305]
    tunnel: w9 -> [w300]
    shift-right: [w291] -> w24
    shift-left: w14 -> [w296]
    tunnel: "notifier" -> [w302]
    tunnel: 100 ("timeout (1 ms)") -> [w298]
    tunnel: w6 -> [w290]
    tunnel: w3 -> [w293]
    tunnel: w5 -> [w292]
    stop <- w297 stop-if-true
    n125 = case shown="No Error" w296 {
      selector: w296 -> [w309 w316]
      tunnel: [w313 _] -> w301
      tunnel: w300 -> [w312 w317]
      tunnel: [w311 w317] -> w299
      tunnel: w298 -> [w310 _]
      tunnel: [w307 "Error" ("message")] -> w295
      tunnel: [w306 w315] -> w294
      frame No Error {
        n126 = Dequeue Element(queue=w312, timeout in ms (-1)=w310, error in (no error)=w309) -> (queue out=w311:refnum<queue>, element=w308:cluster{"message":string, "string":string}, error out=w313:errorcluster)  [unwired: 1 out]
        n127 = Unbundle(w308) -> ("message"=w307:string, "string"=w306:string)
      }
      frame Error {
        n128 = Flatten To String(anything=w316) -> (data string=w315:string)  [unwired: 3 in, 2 out]
      }
    }
    n129 = property class="VI"(reference=w290) -> (reference out=w289:refnum<vi>, "Panel"=w288:refnum<vi>)  [unwired: 1 in, 1 out]
    n130 = Not A Number/Path/Refnum?(number/path/refnum=w302) -> (NaN/Path/Refnum?=w303:bool)
    n131 = case shown="\"\", \"Idle\"" w295 {
      selector: w295 -> [_ _ _ _ _ _ w573 _ _ _ _ w638 _ _ _ _ _ _ _ _ _ _ _ _ _ _ _ _ _ _ _]
      tunnel: w294 -> [_ _ _ _ _ w505 _ _ _ _ _ _ w662 _ _ _ _ w844 w856 w891 w953 w969 w1003 w1022 w1067 w1083 _ w1107 w1138 w1207 w1245]
      tunnel: w301 -> [w319 w326 w356 w419 w443 w506 w577 w584 w598 w615 w628 w640 w670 w698 w766 w803 w823 w845 w855 w885 w962 w973 w1000 w1020 w1064 w1082 w1097 w1108 w1143 w1208 w1246]
      tunnel: [w319 w330 w352 w417 w436 w508 w570 w578 w599 w606 w628 w642 w660 w703 w769 w806 w823 w830 w865 w892 w948 w966 w987 w1025 w1059 w1085 w1097 w1102 w1146 w1196 w1242] -> w291
      tunnel: [w318 w341 w351 w428 w439 w507 w571 w594 w604 w624 w627 w631 w676 w718 w773 w805 w822 w853 w860 w890 w963 w967 w1005 w1029 w1062 w1087 w1096 w1100 w1147 w1214 w1240] -> w304
      tunnel: w305 -> [w318 w339 w351 w412 w440 w507 w571 w594 w604 w624 w627 w631 w675 w719 w774 w808 w822 w852 w861 w890 w960 w965 w1006 w1029 w1061 w1084 w1096 w1101 w1148 w1214 w1241]
      tunnel: w299 -> [_ w329 w359 w424 w438 w498 _ w587 w596 w614 _ w635 w671 w701 _ _ _ w826 _ w889 _ _ _ w1026 w1051 w1077 _ _ w1150 w1199 w1239]
      tunnel: w302 -> [_ w336 w357 w414 w445 w496 _ _ _ _ _ _ w672 _ _ _ _ _ _ w883 _ _ w991 _ _ w1069 _ _ _ w1209 _]
      tunnel: w303 -> [_ w334 w358 w413 w444 w495 _ _ _ _ _ _ w663 w699 _ _ _ _ _ _ _ _ w992 _ _ _ _ _ _ w1197 _]
      tunnel: [_ _ _ _ _ _ _ _ _ TRUE ("Exit") _ _ _ _ _ _ _ _ _ _ _ _ _ _ _ _ _ _ _ _ _] -> w297
      tunnel: w289 -> [_ _ w363 w421 w441 _ w568 _ _ w605 _ _ _ _ _ _ _ _ _ _ _ _ w993 _ _ _ _ _ _ _ _]
      tunnel: w293 -> [_ w323 _ w408 w442 _ _ _ _ _ _ _ _ _ _ _ _ w824 w854 w886 w946 w964 w996 _ _ w1073 _ _ _ w1210 w1238]
      tunnel: w292 -> [_ _ _ _ _ _ _ _ _ w620 _ _ _ _ _ _ _ _ _ _ _ _ w995 w1019 _ _ _ _ _ _ _]
      tunnel: w288 -> [_ _ _ _ _ _ _ w592 _ w619 _ _ _ _ _ _ _ _ _ _ _ _ _ w1018 _ _ _ _ _ _ _]
      frame "------------Generic Operations------------" {
        # "Dummy case to add a seperation in the Case Structure menu"
      }
      frame "Read INI" {
        w327 = "Test Config.ini"
        n132 = Bundle("Initialize", "") -> (w332:cluster{string, string})  [unwired: 1 in]
        n133 = Enqueue Element(queue=w329, element=w332, error in (no error)=w326) -> (error out=w325:errorcluster)  [unwired: 1 in, 2 out]
        n134 = case shown="False" w334 {
          tunnel: w336 -> [w348 _]
          tunnel: w325 -> [w345 w349]
          tunnel: [w344 w349] -> w322
          tunnel: w327 -> [w343 _]
          frame False {
            n135 = Bundle("notification"="Read INI", w343) -> (w346:cluster{"notification":string, string})  [unwired: 1 in]
            n136 = Send Notification(notification=w346, notifier=w348, error in (no error)=w345) -> (error out=w344:errorcluster)  [unwired: 1 out]
          }
          frame True {
          }
        }
        n137 = invoke class="Tree (strict)" method="Edit Tree Items.Delete"(reference=w323, "Delete Children"=TRUE ("Delete Children?")) -> (reference out=w321:refnum<vi>)  [unwired: 3 in, 4 out]
        n138 = call <vilib>:"Application Directory.vi"() -> ("Application Directory"=w338:path)
        n139 = Build Path(base path=w338, name or relative path=w327) -> (appended path=w342:path)
        n140 = invoke class="Tree (strict)" method="Custom Item Symbols.Revert Symbols"(reference=w321, error in=w322) -> (error out=w320:errorcluster)  [unwired: 1 in, 2 out]
        n141 = call "Read INI File.vi"("INI File"=w342) -> ("File paths"=w337:T4, "INI refnum"=w340:T6)  [unwired: 8 in, 1 out]
        n142 = Unbundle By Name(w337) -> ("Error Log"=w335:path)
        n143 = call "Log Error.vi"("Error In"=w320, "Log Path"=w335) -> ("Error Out"=w330:errorcluster, "Log refnum out"=w328:refnum<file>)  [unwired: 8 in]
        n144 = Bundle By Name(cluster=w339, "INI file ref"=w340, "paths"=w337, "Error Log"=w328) -> (w341:T1)
      }
      frame "Initialize" {
        # "Note: LabVIEW Global Variables are safe to use here because they are only written to at the start of the application and clearing them when finalizing shutdown. \n \nNote: You can right click a global and select Find » Global References to view all of the locations where a variable is accessed."
        n145 = case shown="False" w358 {
          tunnel: w357 -> [w369 _]
          tunnel: w356 -> [w366 w370]
          tunnel: [w365 w370] -> w355
          frame False {
            n146 = Bundle("notification"="Initialize", "") -> (w367:cluster{"notification":string, string})  [unwired: 1 in]
            n147 = Send Notification(notification=w367, notifier=w369, error in (no error)=w366) -> (error out=w365:errorcluster)  [unwired: 1 out]
          }
          frame True {
          }
        }
        n148 = Unbundle By Name(w351) -> ("standard events.Quit App"=w350:refnum<user-event>)
        n149 = stacked-sequence {
          tunnel: w363 -> [_ _ w399]
          tunnel: w350 -> [_ _ w398]
          tunnel: w359 -> [_ _ w394]
          tunnel: w355 -> [_ _ w393]
          tunnel: [_ _ w389] -> w354
          frame #0 {
            n150 = global write "Control Globals.vi" "Application Manager"("Application Manager") -> ()
            n151 = global write "Control Globals.vi" "SequenceFileView Manager"("SequenceFileView Manager") -> ()
            n152 = global write "Control Globals.vi" "ExecutionView Manager"("ExecutionView Manager") -> ()
            n153 = global write "Control Globals.vi" "Open Sequence File Btn"("Open Sequence File Btn") -> ()
            n154 = global write "Control Globals.vi" "Close Sequence File Btn"("Close Sequence File Btn") -> ()
            n155 = global write "Control Globals.vi" "Sequence Files ComboBox"("Sequence Files ComboBox") -> ()
            n156 = global write "Control Globals.vi" "Sequences ComboBox"("Sequences ComboBox") -> ()
            n157 = global write "Control Globals.vi" "Run Selected Sequence Btn"("Run Selected Sequence Btn") -> ()
            n158 = global write "Control Globals.vi" "Entry Point 1 Btn"("Entry Point 1 Btn") -> ()
            n159 = global write "Control Globals.vi" "Entry Point 2 Btn"("Entry Point 2 Btn") -> ()
          }
          frame #1 {
            n160 = global write "Control Globals.vi" "Executions ComboBox"("Executions ComboBox") -> ()
            n161 = global write "Control Globals.vi" "Execution View"("Execution View") -> ()
            n162 = global write "Control Globals.vi" "Report Viewer"("Report Viewer") -> ()
            n163 = global write "Control Globals.vi" "Break/Resume Btn"("Break/Resume Btn") -> ()
            n164 = global write "Control Globals.vi" "Terminate/Restart Btn"("Terminate/Restart Btn") -> ()
            n165 = global write "Control Globals.vi" "Close Executions Btn"("Close Executions Btn") -> ()
            n166 = global write "Control Globals.vi" "Terminate All Btn"("Terminate All Btn") -> ()
          }
          frame #2 {
            n167 = global write "Control Globals.vi" "Top level VI"(w399) -> ()
            n168 = global write "Control Globals.vi" "Quit Application Event"(w398) -> ()
            n169 = Bundle("Start Application", "") -> (w397:cluster{string, string})  [unwired: 1 in]
            n170 = Enqueue Element(queue=w394, element=w397, error in (no error)=w393) -> (error out=w392:errorcluster)  [unwired: 1 in, 2 out]
            n171 = property on="TS Pane" class="Bool (strict)"(error in=w392, "Val(Sgnl)"=FALSE ("Value (Signaling)")) -> (error out=w390:errorcluster)  [unwired: 1 in, 1 out]
            n172 = property on="Record" class="Bool (strict)"(error in=w390, "Value"=FALSE ("Record")) -> (error out=w389:errorcluster)  [unwired: 1 in, 1 out]
          }
        }
        n173 = call "Get Engine Reference.vi"("error in (no error)"=w354) -> ("error out"=w360:errorcluster)  [unwired: 10 in]
        n174 = call "Configure Application Manager.vi"("error in (no error)"=w360) -> ("error out"=w362:errorcluster)  [unwired: 10 in]
        n175 = call "Configure SequenceFileView Manager.vi"("error in (no error)"=w362) -> ("error out"=w361:errorcluster)  [unwired: 10 in]
        n176 = call "Configure ExecutionView Manager.vi"("error in"=w361) -> ("error out"=w353:errorcluster)  [unwired: 10 in]
        n177 = call "Configure Event Callback.vi"("error in (no error)"=w353) -> ("error out"=w352:errorcluster)  [unwired: 10 in]
      }
      frame "Start Application" {
        w420 = TRUE ("Front Panel Window:Is Frontmost")
        n178 = Unbundle By Name(w412) -> ("paths.Glyphs"=w411:path)
        n179 = Bundle("New", "") -> (w427:cluster{string, string})  [unwired: 1 in]
        n180 = property class="VI"(reference=w421, "Front Panel.TitleBarVis"=w420, "Front Panel.IsFrontmost"=w420) -> (reference out=w423:refnum<vi>, error out=w422:errorcluster)  [unwired: 1 in]
        n181 = Enqueue Element(queue=w424, element=w427, error in (no error)=w419) -> (error out=w415:errorcluster)  [unwired: 1 in, 2 out]
        n182 = case shown="False" w413 {
          tunnel: w414 -> [w434 _]
          tunnel: w415 -> [w431 w435]
          tunnel: [w430 w435] -> w409
          frame False {
            n183 = Bundle("notification"="Start", "") -> (w432:cluster{"notification":string, string})  [unwired: 1 in]
            n184 = Send Notification(notification=w432, notifier=w434, error in (no error)=w431) -> (error out=w430:errorcluster)  [unwired: 1 out]
          }
          frame True {
          }
        }
        n185 = invoke class="VI" method="Default Vals.Reinit All"(reference=w423, error in=w422) -> (reference out=w404:refnum<vi>)  [unwired: 1 in, 2 out]
        n186 = call "create glyph manager.vi"("error in"=w409, "tree ref (for default symbols)"=w408) -> ("error out"=w403:errorcluster, "glyph manager"=w402:T21)  [unwired: 8 in]
        n187 = call "update tree control.vi"("error in"=w403, "tree reference"=w408, "glyph manager in"=w402) -> ("error out"=w400:errorcluster, "glyph manager out"=w401:T21)  [unwired: 7 in]
        n188 = call "add search path.vi"("error in"=w400, "search path"=w411, "glyph manager in"=w401) -> ("error out"=w407:errorcluster, "glyph manager out"=w410:T21)  [unwired: 7 in]
        n189 = Current VI's Menubar() -> (w406:refnum<k9>)
        n190 = global read "Control Globals.vi" "Application Manager"() -> (w416:refnum<k7>)
        n191 = call "MenuOptions.vi"("VI ref"=w404, "menu ref in"=w406) -> ("menu ref out"=w405:refnum<k9>)  [unwired: 8 in, 1 out]
        n192 = call <vilib>:"TestStand - Set TestStand Application Window.vi"("error in (no error)"=w407, "VI Refnum (Caller's Refnum)"=w404, "Application Manager"=w416) -> ("error out"=w418:errorcluster)  [unwired: 8 out]
        n193 = invoke class="IApplicationMgr" method="Start"(reference=w416, error in=w418) -> (error out=w417:errorcluster)  [unwired: 1 in, 2 out]
        n194 = Bundle By Name(cluster=w412, "glyph manager"=w410, "menu"=w405) -> (w428:T1)
      }
      frame "", "Idle" {
        n195 = case shown="True" w444 {
          tunnel: w445 -> [_ _]
          tunnel: w443 -> [w447 w460]
          tunnel: [w447 w456] -> w437
          tunnel: w442 -> [_ w449]
          tunnel: w441 -> [_ w458]
          tunnel: w440 -> [w446 w461]
          tunnel: [w446 w461] -> w439
          tunnel: w438 -> [_ w455]
          frame False {
          }
          frame True {
            n196 = Unbundle By Name(w461) -> ("current path"=w462:path, "root"=w452:T2, "Record"=w451:bool, "tdms file"=w448:refnum<k34>)
            n197 = property class="Tree (strict)"(reference=w449, error in=w460) -> (reference out=w467:refnum<vi>, error out=w459:errorcluster, "All Tags"=w469:string[], "NumRows"=w466:u32)
            n198 = property class="NISE_CEF_Node"(reference=w452) -> ("DataAccess:Children"=w454:refnum<data-value>[])  [unwired: 1 in, 2 out]
            n199 = Array Size(array=w469) -> (size(s)=w465:i32)
            n200 = To Unsigned Long Integer(number=w465) -> (unsigned 32bit integer=w468:u32)
            n201 = Path To String(path=w462) -> (string=w463:string)
            n202 = Greater Or Equal?(x=w468, y=w466) -> (x >= y?=w464:bool)
            n203 = property class="VI"(reference=w458, "Front Panel.Title"=w463) -> ()  [unwired: 1 in, 2 out]
            n204 = Index Array(array=w454) -> (element=w453:refnum<data-value>)  [unwired: 1 in]
            n205 = property class="Tree (strict)"(reference=w467, error in=w459, "VScrollVis"=w464) -> (error out=w457:errorcluster)  [unwired: 1 out]
            n206 = property class="NISE_CEF_Node"(reference=w453) -> ("DataAccess:Children"=w450:refnum<data-value>[])  [unwired: 1 in, 2 out]
            n207 = case shown="True" w451 {
              tunnel: w457 -> [w470 w478]
              tunnel: [w470 w477] -> w456
              tunnel: w455 -> [_ w476]
              tunnel: w450 -> [_ w475]
              tunnel: w449 -> [_ w474]
              tunnel: w448 -> [_ w473]
              frame False {
              }
              frame True {
                n208 = for {
                  tunnel: w475 -> [w484] mode=indexing
                  shift-right: [w482] -> w477
                  shift-left: w478 -> [w483]
                  tunnel: w474 -> [w481]
                  tunnel: w476 -> [w480]
                  tunnel: w473 -> [w479]
                  n209 = in-place {
                    in-place-border: w483 -> [w488]
                    in-place-border: [w489] -> w482
                    in-place-border: w481 -> [w491]
                    in-place-border: w480 -> [w486]
                    in-place-border: w479 -> [w485]
                    n210 = in-place-dvr #4(w484) -> (w492:refnum<class "CEF_Node.lvclass">)  [unwired: 1 out]
                    n211 = call-dynamic "MenuHandler.vi"("tree control"=w491, "main queue"=w486, "error in"=w488, "parameters"=w485, "menu string"="Record", "CEF_Node in"=w492) -> ("error out"=w489:errorcluster, "CEF_Node out"=w490:refnum<class "CEF_Node.lvclass">)  [unwired: 2 in, 2 out]
                    n212 = in-place-dvr #4(w490) -> ()  [unwired: 2 out]
                  }
                }
                n213 = call "Timing FGV.vi"("Timer Mode"=T19."Read Time") -> ("Elapsed Time (s.ms)"=→"Time":dbl)  [unwired: 8 in, 2 out]
              }
            }
          }
        }
        n214 = call <vilib>:"Unset Busy.vi"("error in (no error)"=w437) -> ("error out"=w436:errorcluster)  [unwired: 10 in]
      }
      frame "Error" {
        n215 = Unflatten From String(type=errorcluster {"status"=FALSE, "code"=0, "source"=""} ("error out"), binary string=w505, error in (no error)=w506) -> (value=w503:errorcluster)  [unwired: 2 in, 2 out]
        n216 = Get Date/Time In Seconds() -> (seconds since 1Jan1904=w511:timestamp)
        n217 = Unbundle By Name(w503) -> ("code"=w494:i32)
        n218 = Format Date/Time String(time format string (%c)="%H:%M:%S", seconds (now)=w511) -> (date/time string=w502:string)  [unwired: 1 in]
        n219 = Unbundle By Name(w507) -> ("Error Log"=w501:refnum<file>)
        n220 = case shown="1, 91, 1556, 5001" w494 {
          tunnel: w503 -> [w518 w520 w523 w530 w533 w535 w540 w548 w549 w554 w559]
          tunnel: [w519 w521 w525 w529 w532 w536 w538 w545 w550 w552 w557] -> w493
          tunnel: w498 -> [_ _ _ _ _ _ _ _ _ _ w567]
          tunnel: [w518 _ w522 w528 w531 w534 w537 _ w549 w551 w558] -> w497
          tunnel: w496 -> [_ _ _ _ _ _ _ _ _ _ w560]
          tunnel: w495 -> [_ _ _ _ _ _ _ _ _ _ _]
          frame 538504, 538505 {
            n221 = Unbundle By Name(w518) -> ("source"=w519:string)
          }
          frame Default {
            n222 = call <vilib>:"Simple Error Handler.vi"("error in (no error)"=w520) -> ()  [unwired: 4 in, 5 out]
            n223 = Unbundle By Name(w520) -> ("source"=w521:string)
          }
          frame -2147220623, -2147220621, -2147220364, 56, 63, 537053 {
            n224 = Unbundle By Name(w523) -> ("source"=w527:string)
            n225 = Concatenate Strings(w527, "\n", "*Note : Problem communicating with remote device.  Make sure a valid device is selected and that the IP address is correct.\n" ("message")) -> (w525:string)
            n226 = Bundle By Name(cluster=w523, "source"=w525) -> (w522:errorcluster)
          }
          frame 1000 {
            w529 = "Invoke error : Abort VI at Subpanel." ("message")
            n227 = Bundle By Name(cluster=w530, "source"=w529) -> (w528:errorcluster)
          }
          frame 1003 {
            w532 = "Dev Error: The Ui.vi for the selected class is broken." ("message")
            n228 = Bundle By Name(cluster=w533, "source"=w532) -> (w531:errorcluster)
          }
          frame 1, 91, 1556, 5001 {
            w536 = "Make sure Variant to data." ("message")
            n229 = Bundle By Name(cluster=w535, "source"=w536) -> (w534:errorcluster)
          }
          frame 15550 {
            n230 = Unbundle By Name(w540) -> ("source"=w542:string)
            n231 = Concatenate Strings(w542, "\n", "*Note : The System does not yet have a configuration to download. Create or open a configuration and download it to the System" ("message")) -> (w538:string)
            n232 = Bundle By Name(cluster=w540, "source"=w538) -> (w537:errorcluster)
          }
          frame -375006, 537549, 538500 {
            n233 = Unbundle By Name(w548) -> ("source"=w544:string)
            n234 = Concatenate Strings(w544, "\n", "*Note : Invalid configuration when opening config file. Check out if it existed or both tags and class names are correct." ("message")) -> (w545:string)
            n235 = Bundle By Name(cluster=w548, "source"=w545) -> (w547:errorcluster)
            n236 = call <vilib>:"Simple Error Handler.vi"("error in (no error)"=w547) -> ()  [unwired: 4 in, 5 out]
          }
          frame 42..44 {
            # "42 : Node Invalid\n43 : Engine unInitialized\n44 : JSON to LVobject"
            n237 = Unbundle By Name(w549) -> ("source"=w550:string)
          }
          frame 402840 {
            # "check out configuration class"
            n238 = Unbundle By Name(w554) -> ("source"=w556:string)
            n239 = Concatenate Strings(w556, "\n", "JSON is blank because identifier unknown to unwrap or wrap " ("message")) -> (w552:string)
            n240 = Bundle By Name(cluster=w554, "source"=w552) -> (w551:errorcluster)
          }
          frame -17006 {
            w557 = "starting application.\nPlease restart LabVIEW program" ("format string")
            # "Teststand UI starting Error"
            n241 = Bundle("Message Name"="Close?", "") -> (w564:cluster{"Message Name":string, string})  [unwired: 1 in]
            n242 = Bundle("notification"="Done", variant) -> (w563:cluster{"notification":string, variant})  [unwired: 1 in]
            n243 = Enqueue Element(queue=w567, element=w564) -> ()  [unwired: 2 in, 3 out]
            n244 = Send Notification(notification=w563, notifier=w560) -> ()  [unwired: 1 in, 2 out]
            n245 = Bundle By Name(cluster=w559, "source"=w557) -> (w558:errorcluster)
          }
        }
        n246 = call "one shot error.vi"("error in"=w497) -> ()  [unwired: 11 in]
        n247 = Format Into String(format string="%1$s\t%2$d\t%3$s\n", w502, w494, w493) -> (resulting string=w509:string)  [unwired: 2 in, 1 out]
        n248 = Not A Number/Path/Refnum?(number/path/refnum=w501) -> (NaN/Path/Refnum?=w500:bool)
        n249 = case shown="False" w500 {
          tunnel: w509 -> [w516 _]
          tunnel: [w515 w517] -> w508
          tunnel: w501 -> [w514 _]
          tunnel: errorcluster {"status"=FALSE, "code"=0, "source"=""} ("error in") -> [w513 w517]
          frame False {
            n250 = Write to Text File(file (use dialog)=w514, text=w516, error in=w513) -> (error out=w515:errorcluster)  [unwired: 1 in, 2 out]
          }
          frame True {
          }
        }
      }
      frame "Missing Message Handler", Default {
        # "Call this case if a message is received that is not handled by any other case. Typically this is a programming error as a result of a typo or unhandled message/missing message handler."
        n251 = property class="VI"(reference=w568) -> (reference out=w569:refnum<vi>, "Name"=w575:string)  [unwired: 1 in, 1 out]
        n252 = Format Into String(format string="DevError: Missing message handler for '%s\" message." ("message"), w573) -> (resulting string=w572:string)  [unwired: 2 in, 1 out]
        n253 = call <vilib>:"Unset Busy.vi"("VI reference (current VI)"=w569) -> ()  [unwired: 10 in, 1 out]
        n254 = call "CEF_error generator.vi"("error in"=w577, "source"=w575, "append error message"=w572, "error code (0)"=538505) -> ("error out"=w570:errorcluster)  [unwired: 5 in]
      }
      frame "Close" {
        w582 = FALSE  # Reset
        n255 = Flatten To String(anything=w582, error in (no error)=w584) -> (data string=w581:string, error out=w583:errorcluster)  [unwired: 2 in, 1 out]
        n256 = Bundle("Control Engines", "data string"=w581) -> (w585:cluster{string, "data string":string})  [unwired: 1 in]
        n257 = Enqueue Element(queue=w587, element=w585, error in (no error)=w583) -> (queue out=w580:refnum<queue>, error out=w588:errorcluster)  [unwired: 1 in, 1 out]
        n258 = Bundle("Write INI File", "") -> (w591:cluster{string, string})  [unwired: 1 in]
        n259 = Enqueue Element(queue=w580, element=w591, error in (no error)=w588) -> (error out=w579:errorcluster)  [unwired: 1 in, 2 out]
        n260 = property class="Pnl"(reference=w592, error in=w579, "DeferPanUpdts"=TRUE ("Defer Panel Updates")) -> (error out=w578:errorcluster)  [unwired: 1 out]
      }
      frame "Write INI File" {
        n261 = Unbundle By Name(w604) -> ("INI file ref"=w595:T6, "paths"=w603:T4)
        n262 = Bundle("Shutdown", "") -> (w602:cluster{string, string})  [unwired: 1 in]
        n263 = Enqueue Element(queue=w596, element=w602, error in (no error)=w598) -> (error out=w597:errorcluster)  [unwired: 1 in, 2 out]
        n264 = call "Write INI File.vi"("error in"=w597, "File path"=w603, "INI refnum"=w595) -> ("error out"=w599:errorcluster)  [unwired: 8 in]
      }
      frame "Shutdown" {
        # "close root DVR"
        n265 = Release Queue(queue=w614, error in (no error)=w615) -> (error out=w611:errorcluster)  [unwired: 1 in, 2 out]
        n266 = property class="Pnl"(reference=w619, "DeferPanUpdts"=FALSE ("Defer Panel Updates")) -> ()  [unwired: 1 in, 2 out]
        n267 = global read "Control Globals.vi" "TestStand Engine"() -> (w612:refnum<k7>)
        n268 = Unbundle By Name(w624) -> ("root"=w622:T2, "Error Log"=w623:refnum<file>, "standard events"=w618:T3)
        n269 = Close Reference(reference=w612, error in (no error)=w611) -> (error out=w610:errorcluster)
        n270 = global read "Control Globals.vi" "Event Callback"() -> (w613:refnum<k27>)
        n271 = Unregister For Events(event registration refnum=w613, error in=w610) -> (error out=w609:errorcluster)
        n272 = call "ClearStandardEvents.vi"("error in"=w609, "standard events"=w618, "sub panel ref in"=w620) -> ("error out"=w616:errorcluster)  [unwired: 8 in]
        n273 = Close File(refnum=w623, error in=w616) -> (error out=w617:errorcluster)  [unwired: 1 out]
        n274 = call "CloseNode.vi"("error in"=w617, "node ref"=w622) -> ("error out"=w607:errorcluster)  [unwired: 9 in]
        n275 = disable-structure shown="RUN_TIME_ENGINE==True" {
          disable-tunnel: w607 -> [w625 w626]
          disable-tunnel: [w625 w626] -> w606
          disable-tunnel: w605 -> [_ _]
          frame condition #0 (active) {
          }
          frame condition #1 {
            n276 = Quit LabVIEW() -> ()  [unwired: 1 in]
          }
        }
      }
      frame "------------Menu Operations--------------" {
        # "Dummy case to add a seperation in the Case Structure menu"
      }
      frame "Close?", "New?", "Open?" {
        n277 = Unbundle By Name(w631) -> ("current path"=w630:path, "unsaved changes"=w632:bool, "repository"=w634:refnum<class "CEF_Repository.lvclass">, "root"=w633:T2)
        n278 = case shown="True" w632 {
          tunnel: w640 -> [w651 w659]
          tunnel: [w651 w652] -> w641
          tunnel: [TRUE ("Cancelled") w654] -> w639
          tunnel: w634 -> [_ w656]
          tunnel: w633 -> [_ w657]
          tunnel: w630 -> [_ w653]
          frame False {
            # "If there is nothing to save Go do Action"
          }
          frame True {
            n279 = call-dynamic "ReadTree.vi"("error in"=w659, "root"=w657, "CEF_Repository in"=w656) -> ("error out"=w658:errorcluster, "CEF_Repository out"=w655:refnum<class "CEF_Repository.lvclass">)  [unwired: 7 in]
            n280 = call "SaveDialog.vi"("error in"=w658, "current path"=w653, "repository"=w655) -> ("error out"=w652:errorcluster, "Done?"=w654:bool)  [unwired: 6 in, 1 out]
          }
        }
        n281 = Search and Replace String(input string=w638, search string="?", replace string="") -> (result string=w629:string)  [unwired: 5 in, 3 out]
        n282 = case shown="True" w639 {
          tunnel: [w643 w648] -> w642
          tunnel: w641 -> [w643 w649]
          tunnel: w635 -> [_ w647]
          tunnel: w629 -> [_ w646]
          frame False {
          }
          frame True {
            n283 = Bundle("result string"=w646, "") -> (w644:cluster{"result string":string, string})  [unwired: 1 in]
            n284 = Enqueue Element(queue=w647, element=w644, error in (no error)=w649) -> (error out=w648:errorcluster)  [unwired: 1 in, 2 out]
          }
        }
      }
      frame "New" {
        n285 = case shown="False" w663 {
          tunnel: w672 -> [w689 _]
          tunnel: w671 -> [w685 w693]
          tunnel: w670 -> [w683 w696]
          tunnel: [w677 w695] -> w668
          tunnel: [w679 path "" ("Configuration file")] -> w664
          tunnel: w675 -> [w686 _]
          tunnel: w662 -> [_ _]
          frame False {
            n286 = Unbundle By Name(w686) -> ("paths.Configuration"=w679:path)
            n287 = Bundle("notification"="Open", "") -> (w684:cluster{"notification":string, string})  [unwired: 1 in]
            n288 = Enqueue Element(queue=w685, element=w684, error in (no error)=w683) -> (error out=w680:errorcluster)  [unwired: 1 in, 2 out]
            n289 = Path To String(path=w679) -> (string=w678:string)
            n290 = Bundle("notification"="Open Config", w678) -> (w687:cluster{"notification":string, string})  [unwired: 1 in]
            n291 = Send Notification(notification=w687, notifier=w689, error in (no error)=w680) -> (error out=w677:errorcluster)  [unwired: 1 out]
          }
          frame True {
            n292 = Bundle("PopulateTree", "") -> (w690:cluster{string, string})  [unwired: 1 in]
            n293 = Enqueue Element(queue=w693, element=w690, error in (no error)=w696) -> (error out=w695:errorcluster)  [unwired: 1 in, 2 out]
          }
        }
        n294 = Unbundle By Name(w675) -> ("paths.Plugin"=w669:path)
        n295 = call-dynamic "Initialize.vi"("error in"=w668, "path"=w669, "CEF_Repository in"=refnum<class "CEF_HierarchyRepo.lvclass"> refnum ("CEF.lvlibp:CEF_HierarchyRepo.lvclass")) -> ("error out"=w673:errorcluster, "CEF_Repository out"=w665:refnum<class "CEF_HierarchyRepo.lvclass">)  [unwired: 7 in]
        n296 = call-dynamic "Initialize.vi"("error in"=w673, "CEF_Serialize node in"=refnum<class "System.lvclass"> refnum ("System.lvlibp:System")) -> ("error out"=w660:errorcluster, "data value reference"=w667:refnum<data-value>)  [unwired: 7 in, 1 out]
        n297 = Bundle By Name(cluster=w675, "unsaved changes"=FALSE, "current path"=w664, "repository"=w665, "root"=w667) -> (w676:T1)
      }
      frame "Open" {
        n298 = Unbundle By Name(w719) -> ("unsaved changes"=w714:bool, "root"=w713:T2, "repository"=w704:refnum<class "CEF_Repository.lvclass">, "current path"=w705:path, "paths.Configuration"=w708:path)
        n299 = case shown="True" w699 {
          tunnel: w698 -> [w720 w722]
          tunnel: [w720 w721] -> w697
          frame False {
          }
          frame True {
            n300 = invoke class="VI" method="FP.Open"(error in=w722) -> (error out=w721:errorcluster)  [unwired: 4 in, 4 out]
          }
        }
        n301 = Equal?(x=w708, y=path "" ("f")) -> (x = y?=w709:bool)
        n302 = Not(x=w709) -> (.not. x?=w711:bool)
        n303 = Not(x=w699) -> (.not. x?=w700:bool)
        n304 = And(x=w711, y=w700) -> (x .and. y?=w702:bool)
        n305 = case shown="False" w702 {
          tunnel: [w725 w726] -> w717
          tunnel: [w724 _] -> w716
          tunnel: w708 -> [w723 w726]
          frame False {
            n306 = call "FileDialog.vi"("start path"=w723) -> ("cancelled"=w724:bool, "selected path"=w725:path)  [unwired: 8 in, 1 out]
          }
          frame True {
          }
        }
        n307 = case shown="False" w716 {
          tunnel: [w728 w761] -> w703
          tunnel: w697 -> [w741 w761]
          tunnel: w713 -> [w736 w762]
          tunnel: [w734 w763] -> w707
          tunnel: w717 -> [w737 w763]
          tunnel: w714 -> [_ w764]
          tunnel: [FALSE ("unsaved changes") w764] -> w715
          tunnel: [w735 w762] -> w712
          tunnel: w705 -> [w733 _]
          tunnel: w704 -> [w731 w760]
          tunnel: [w732 w760] -> w706
          tunnel: w700 -> [w730 _]
          tunnel: w701 -> [w729 _]
          frame False {
            n308 = call-dynamic "Open.vi"("error in"=w741, "file path"=w737, "CEF_Repository in"=w731) -> ("error out"=w739:errorcluster, "invalid?"=w740:bool, "CEF_Repository out"=w738:refnum<class "CEF_Repository.lvclass">)  [unwired: 6 in]
            n309 = case shown="False" w740 {
              tunnel: [w752 w759] -> w732
              tunnel: [w743 w755] -> w728
              tunnel: [w749 w758] -> w735
              tunnel: w738 -> [w751 w759]
              tunnel: w739 -> [w748 w755]
              tunnel: w737 -> [w750 _]
              tunnel: w736 -> [_ w758]
              tunnel: [w750 w757] -> w734
              tunnel: w733 -> [_ w757]
              tunnel: w730 -> [w746 _]
              tunnel: [w744 w753] -> w727
              frame False {
                n310 = call-dynamic "WriteTree.vi"("error in"=w748, "CEF_Repository in"=w751) -> ("error out"=w743:errorcluster, "root"=w749:refnum<data-value>, "CEF_Repository out"=w752:refnum<class "CEF_Repository.lvclass">)  [unwired: 7 in]
                n311 = Flatten To String(anything=w746) -> (data string=w745:string)  [unwired: 3 in, 2 out]
                n312 = Bundle("Control Engines", "data string"=w745) -> (w744:cluster{string, "data string":string})  [unwired: 1 in]
              }
              frame True {
                n313 = Bundle("notification"="PopulateTree", "") -> (w753:cluster{"notification":string, string})  [unwired: 1 in]
              }
            }
            n314 = Enqueue Element(queue=w729, element=w727) -> ()  [unwired: 2 in, 3 out]
          }
          frame True {
          }
        }
        n315 = Bundle By Name(cluster=w719, "unsaved changes"=w715, "root"=w712, "repository"=w706, "current path"=w707, "paths.Configuration"=w707) -> (w718:T1)
      }
      frame "Save" {
        n316 = Unbundle By Name(w774) -> ("current path"=w775:path, "repository"=w765:refnum<class "CEF_Repository.lvclass">, "root"=w776:T2)
        n317 = Empty String/Path?(string/path=w775) -> (empty?=w777:bool)
        n318 = Not A Number/Path/Refnum?(number/path/refnum=w775) -> (NaN/Path/Refnum?=w778:bool)
        n319 = call-dynamic "ReadTree.vi"("error in"=w766, "root"=w776, "CEF_Repository in"=w765) -> ("error out"=w772:errorcluster, "CEF_Repository out"=w771:refnum<class "CEF_Repository.lvclass">)  [unwired: 7 in]
        n320 = Or(x=w777, y=w778) -> (x .or. y?=w779:bool)
        n321 = case shown="True" w779 {
          tunnel: w775 -> [w782 w792]
          tunnel: [w782 w791] -> w767
          tunnel: w772 -> [w784 w786]
          tunnel: w771 -> [w783 w789]
          tunnel: [w780 w788] -> w770
          tunnel: [w781 w787] -> w769
          frame False {
            # "unchanged file path"
            n322 = call-dynamic "Save.vi"("error in"=w784, "file path"=w782, "CEF_Repository in"=w783) -> ("error out"=w781:errorcluster, "CEF_Repository out"=w780:refnum<class "CEF_Repository.lvclass">)  [unwired: 7 in]
          }
          frame True {
            # "Empthy path, Not a Path, and changed"
            n323 = call "FileDialog.vi"("error in"=w786, "start path"=w792) -> ("error out"=w785:errorcluster, "cancelled"=w793:bool, "selected path"=w790:path)  [unwired: 7 in]
            n324 = case shown="False" w793 {
              tunnel: [w796 w801] -> w791
              tunnel: w790 -> [w796 w801]
              tunnel: w785 -> [w798 w799]
              tunnel: w789 -> [w797 w800]
              tunnel: [w795 w800] -> w788
              tunnel: [w794 w799] -> w787
              frame False {
                n325 = call-dynamic "Save.vi"("error in"=w798, "file path"=w796, "CEF_Repository in"=w797) -> ("error out"=w794:errorcluster, "CEF_Repository out"=w795:refnum<class "CEF_Repository.lvclass">)  [unwired: 7 in]
              }
              frame True {
              }
            }
          }
        }
        n326 = Unbundle By Name(w769) -> ("status"=w768:bool)
        n327 = Bundle By Name(cluster=w774, "paths.Configuration"=w767, "current path"=w767, "repository"=w770, "unsaved changes"=w768) -> (w773:T1)
      }
      frame "SaveAs" {
        n328 = Unbundle By Name(w808) -> ("current path"=w809:path, "repository"=w802:refnum<class "CEF_Repository.lvclass">, "root"=w814:T2)
        n329 = call-dynamic "ReadTree.vi"("error in"=w803, "root"=w814, "CEF_Repository in"=w802) -> ("error out"=w811:errorcluster, "CEF_Repository out"=w810:refnum<class "CEF_Repository.lvclass">)  [unwired: 7 in]
        n330 = call "FileDialog.vi"("error in"=w811, "start path"=w809) -> ("error out"=w812:errorcluster, "cancelled"=w813:bool, "selected path"=w804:path)  [unwired: 7 in]
        n331 = case shown="False" w813 {
          tunnel: w804 -> [w817 _]
          tunnel: w812 -> [w819 w820]
          tunnel: w810 -> [w818 w821]
          tunnel: [w816 w821] -> w807
          tunnel: [w815 w820] -> w806
          frame False {
            n332 = call-dynamic "Save.vi"("error in"=w819, "file path"=w817, "CEF_Repository in"=w818) -> ("error out"=w815:errorcluster, "CEF_Repository out"=w816:refnum<class "CEF_Repository.lvclass">)  [unwired: 7 in]
          }
          frame True {
          }
        }
        n333 = Bundle By Name(cluster=w808, "paths.Configuration"=w804, "current path"=w804, "repository"=w807) -> (w805:T1)
      }
      frame "-------TreeControl Operations-----------" {
        # "Dummy case to add a seperation in the Case Structure menu"
      }
      frame "AddNode" {
        n334 = Unbundle By Name(w852) -> ("glyph manager"=w851:T5, "repository"=w838:refnum<class "CEF_Repository.lvclass">)
        n335 = Unflatten From String(type=T8 {"subNode"="", "Node ID"=""} ("input cluster"), binary string=w844, error in (no error)=w845) -> (value=w846:T8, error out=w840:errorcluster)  [unwired: 2 in, 1 out]
        n336 = Unbundle By Name(w846) -> ("Node ID"=w843:string, "subNode"=w834:string)
        n337 = call-dynamic "GetClassPath.vi"("error in"=w840, "class name"=w834, "CEF_Repository in"=w838) -> ("error out"=w836:errorcluster, "class path"=w839:path)  [unwired: 6 in, 1 out]
        n338 = call <vilib>:"Get LV Class Default Value.vi"("error in (no error)"=w836, "class path"=w839) -> ("error out"=w835:errorcluster, "object"=w837:refnum<class>)  [unwired: 8 in]
        n339 = To More Specific Class(target class=refnum<class "CEF_serializable node.lvclass"> refnum ("CEF.lvlibp:CEF_serializable node.lvclass"), reference=w837, error in=w835) -> (specific class reference=w841:refnum<class "CEF_serializable node.lvclass">, error out=w842:errorcluster)
        n340 = call "AddNode.vi"("error in"=w842, "parameters"=w834, "parent node ID"=w843, "CEF_Node in"=w841) -> ("error out"=w850:errorcluster, "summary"=w832:T22)  [unwired: 6 in]
        n341 = call "PopulateTreeSumaryWithGlyphManager.vi"("error in"=w850, "glyph manager"=w851, "summary"=w832, "tree ref in"=w824) -> ("error out"=w831:errorcluster, "glyph manager out"=w848:T21)  [unwired: 6 in]
        n342 = Index Array(array=w832) -> (element=w833:T23)  [unwired: 1 in]
        n343 = Unbundle By Name(w833) -> ("ID"=w827:string)
        n344 = Bundle By Name(cluster=w852, "unsaved changes"=TRUE, "glyph manager"=w848) -> (w853:T1)
        n345 = Bundle("format string"="RefreshNode", "ID"=w827) -> (w825:cluster{"format string":string, "ID":string})  [unwired: 1 in]
        n346 = Enqueue Element(queue=w826, element=w825, error in (no error)=w831) -> (error out=w830:errorcluster)  [unwired: 1 in, 2 out]
      }
      frame "Duplicate" {
        n347 = Unbundle By Name(w861) -> ("glyph manager"=w858:T5)
        n348 = call "IDtoNode.vi"("error in"=w855, "ID"=w856) -> ("error out"=w863:errorcluster, "invalid Id"=w862:bool, "node ref"=w864:refnum<data-value>)  [unwired: 7 in]
        n349 = case shown="False" w862 {
          tunnel: [w876 w878] -> w865
          tunnel: w864 -> [w875 _]
          tunnel: w863 -> [w872 w879]
          tunnel: w858 -> [w868 w882]
          tunnel: [w867 w882] -> w857
          tunnel: w854 -> [w866 _]
          frame False {
            n350 = call "DuplicateNode.vi"("same parent?"=TRUE ("s"), "error in"=w872, "node ref in"=w875) -> ("error out"=w873:errorcluster, "new node ref"=w874:refnum<data-value>)  [unwired: 7 in]
            n351 = call "Summary.vi"("error in"=w873, "node self ref"=w874) -> ("error out"=w870:errorcluster, "summary"=w869:T22)  [unwired: 8 in]
            n352 = call "PopulateTreeSumaryWithGlyphManager.vi"("error in"=w870, "glyph manager"=w868, "summary"=w869, "tree ref in"=w866) -> ("error out"=w876:errorcluster, "glyph manager out"=w867:T21)  [unwired: 6 in]
          }
          frame True {
            n353 = call "CEF_error generator.vi"("error in"=w879, "source"="TSS::Duplicate", "append error message"="Node invalid " ("source"), "error code (0)"=42) -> ("error out"=w878:errorcluster)  [unwired: 5 in]
          }
        }
        n354 = Bundle By Name(cluster=w861, "unsaved changes"=TRUE, "glyph manager"=w857) -> (w860:T1)
      }
      frame "CustomMenuAction" {
        n355 = Unbundle By Name(w890) -> ("standard events.node change"=w887:refnum<user-event>)
        n356 = Match Pattern(string=w891, regular expression=":") -> (before substring=w894:string, after substring=w888:string)  [unwired: 1 in, 2 out]
        n357 = call "IDtoNode.vi"("error in"=w885, "ID"=w888) -> ("error out"=w884:errorcluster, "invalid Id"=w895:bool, "node ref"=w896:refnum<data-value>)  [unwired: 7 in]
        n358 = case shown="False" w895 {
          tunnel: [w908 w942] -> w892
          tunnel: w896 -> [w906 _]
          tunnel: w884 -> [w902 w943]
          tunnel: w894 -> [w909 _]
          tunnel: w886 -> [w907 _]
          tunnel: w889 -> [w904 _]
          tunnel: w887 -> [w900 _]
          tunnel: w883 -> [w897 _]
          frame False {
            n359 = in-place {
              in-place-border: [w939] -> w910
              in-place-border: w909 -> [w935]
              in-place-border: w907 -> [w938]
              in-place-border: [w937] -> w905
              in-place-border: w904 -> [w931]
              in-place-border: [w935] -> w903
              in-place-border: w902 -> [w934]
              in-place-border: [w933] -> w901
              in-place-border: w900 -> [w932]
              in-place-border: [w932] -> w899
              in-place-border: w897 -> [w930]
              n360 = in-place-dvr #5(w906) -> (w936:refnum<class "CEF_Node.lvclass">)  [unwired: 1 out]
              n361 = call-dynamic "MenuHandler.vi"("tree control"=w938, "main queue"=w931, "error in"=w934, "parameters"=w930, "menu string"=w935, "CEF_Node in"=w936) -> ("error out"=w933:errorcluster, "refresh tree?"=w937:bool, "Unhandled"=w939:bool, "CEF_Node out"=w940:refnum<class "CEF_Node.lvclass">)  [unwired: 2 in]
              n362 = in-place-dvr #5(w940) -> (w898:refnum<data-value>)  [unwired: 1 out]
            }
            n363 = case shown="False" w910 {
              tunnel: w903 -> [_ w921]
              tunnel: [w915 w922] -> w908
              tunnel: w901 -> [w913 w923]
              tunnel: w905 -> [w914 _]
              tunnel: w899 -> [w912 _]
              tunnel: w898 -> [w911 _]
              frame False {
                n364 = case shown="False" w914 {
                  tunnel: [w916 w917] -> w915
                  tunnel: w913 -> [w916 w918]
                  tunnel: w912 -> [_ w920]
                  tunnel: w911 -> [_ w919]
                  frame False {
                  }
                  frame True {
                    # "update EngineMap"
                    n365 = Generate User Event(user event=w920, event data cluster=w919, error in=w918) -> (error out=w917:errorcluster)  [unwired: 1 in, 1 out]
                  }
                }
              }
              frame True {
                n366 = disable-structure shown="Default" {
                  disable-tunnel: w923 -> [w926 w929]
                  disable-tunnel: [w925 w929] -> w922
                  disable-tunnel: w921 -> [w924 _]
                  frame condition #0 {
                    n367 = call "CEF_error generator.vi"("error in"=w926, "source"="TSS::CustomMenuAction", "append error message"=w924, "error code (0)"=538506) -> ("error out"=w925:errorcluster)  [unwired: 5 in]
                  }
                  frame condition #1 (active) {
                  }
                }
              }
            }
          }
          frame True {
            n368 = call "CEF_error generator.vi"("error in"=w943, "source"="TSS:CustomMenuAction", "append error message"="Node invalid " ("source"), "error code (0)"=42) -> ("error out"=w942:errorcluster)  [unwired: 5 in]
          }
        }
      }
      frame "RefreshNode" {
        # "Refreshes the node in the Tree, Sets the save flag to true. This case can be called from the UIs of the nodes"
        n369 = Unbundle By Name(w960) -> ("glyph manager"=w951:T5, "root"=w947:T2)
        n370 = call "IDtoNode.vi"("error in"=w962, "ID"=w953) -> ("error out"=w952:errorcluster, "invalid Id"=w956:bool, "node ref"=w955:refnum<data-value>)  [unwired: 7 in]
        n371 = Select(t=w947, s=w956, f=w955) -> (s? t:f=w954:T2)
        n372 = call "SummaryWithGlyphManager.vi"("error in"=w952, "glyph manager"=w951, "node self ref"=w954) -> ("error out"=w950:errorcluster, "glyph manager out"=w957:T21, "summary"=w949:T22)  [unwired: 6 in]
        n373 = call "RefreshSubTreeWithGlyphManager.vi"("error in"=w950, "glyph manager"=w957, "node information"=w949, "tree ref in"=w946) -> ("error out"=w959:errorcluster, "glyph manager out"=w961:T21, "tree ref out"=w958:refnum<vi>)  [unwired: 5 in]
        n374 = Close Reference(reference=w958, error in (no error)=w959) -> (error out=w948:errorcluster)
        n375 = Bundle By Name(cluster=w960, "glyph manager"=w961) -> (w963:T1)
      }
      frame "RemoveNode" {
        n376 = call "IDtoNode.vi"("error in"=w973, "ID"=w969) -> ("error out"=w972:errorcluster, "invalid Id"=w970:bool, "node ref"=w971:refnum<data-value>)  [unwired: 7 in]
        n377 = case shown="True" w970 {
          tunnel: w972 -> [w975 w982]
          tunnel: w971 -> [w976 _]
          tunnel: [w977 w981] -> w966
          tunnel: w964 -> [w974 _]
          frame False {
            n378 = call "RemoveNode.vi"("error in"=w975, "node"=w976) -> ("error out"=w978:errorcluster, "node ID"=w979:string)  [unwired: 8 in]
            n379 = call "ClearTreeNode.vi"("error in"=w978, "tag"=w979, "tree reference"=w974) -> ("error out"=w977:errorcluster)  [unwired: 8 in]
          }
          frame True {
            n380 = call "CEF_error generator.vi"("error in"=w982, "source"="TSS:RemoveNode", "append error message"="Node invalid " ("source"), "error code (0)"=42) -> ("error out"=w981:errorcluster)  [unwired: 5 in]
          }
        }
        n381 = Bundle By Name(cluster=w965, "unsaved changes"=TRUE) -> (w967:T1)
      }
      frame "PopulateTree" {
        # "Close the Launch Panel, and show the main UI panel"
        n382 = call <vilib>:"Set Busy.vi"("error in (no error)"=w1000) -> ("error out"=w990:errorcluster)  [unwired: 9 in, 1 out]
        n383 = Unbundle By Name(w1006) -> ("root"=w997:T2, "glyph manager"=w994:T5, "standard events.user event"=w1001:refnum<user-event>)
        n384 = case shown="False" w992 {
          tunnel: w991 -> [w1012 _]
          tunnel: w990 -> [w1009 w1013]
          tunnel: [w1008 w1013] -> w989
          frame False {
            n385 = Bundle("notification"="Launched", "") -> (w1010:cluster{"notification":string, string})  [unwired: 1 in]
            n386 = Send Notification(notification=w1010, notifier=w1012, error in (no error)=w1009) -> (error out=w1008:errorcluster)  [unwired: 1 out]
          }
          frame True {
          }
        }
        n387 = call "ClearSubPanel.vi"("error in"=w989, "user event ref"=w1001, "sub panel ref in"=w995) -> ("error out"=w998:errorcluster)  [unwired: 7 in, 1 out]
        n388 = call "SummaryWithGlyphManager.vi"("error in"=w998, "glyph manager"=w994, "node self ref"=w997) -> ("error out"=w985:errorcluster, "glyph manager out"=w999:T21, "summary"=w986:T22)  [unwired: 6 in]
        n389 = case shown="\"\"" w1003 {
          selector: w1003 -> [w1014 _]
          tunnel: w986 -> [_ w1016]
          tunnel: [w1014 w1015] -> w1002
          frame Default {
          }
          frame "" {
            n390 = Index Array(array=w1016) -> (element=w1017:T23)  [unwired: 1 in]
            n391 = Unbundle By Name(w1017) -> ("ID"=w1015:string)
          }
        }
        n392 = property class="Tree (strict)"(reference=w996, "Val(Sgnl)"=w1002) -> (reference out=w988:refnum<vi>)  [unwired: 1 in, 1 out]
        n393 = call "RefreshEntireTreeWithGlyphManager.vi"("calling VI"=w993, "error in"=w985, "glyph manager"=w999, "array"=w986, "tree ref in"=w988) -> ("error out"=w987:errorcluster, "glyph manager out"=w1004:T21)  [unwired: 5 in]
        n394 = Bundle By Name(cluster=w1006, "glyph manager"=w1004) -> (w1005:T1)
      }
      frame "ActivateNode" {
        n395 = Unbundle By Name(w1029) -> ("standard events"=w1023:T3)
        n396 = property class="Pnl"(reference=w1018, "DeferPanUpdts"=TRUE ("Defer Panel Updates")) -> (reference out=w1021:refnum<vi>)  [unwired: 1 in, 1 out]
        n397 = call "IDtoNode.vi"("error in"=w1020, "ID"=w1022) -> ("error out"=w1027:errorcluster, "invalid Id"=w1030:bool, "node ref"=w1028:refnum<data-value>)  [unwired: 7 in]
        n398 = case shown="False" w1030 {
          tunnel: w1028 -> [w1041 _]
          tunnel: [w1035 w1046] -> w1025
          tunnel: w1027 -> [w1033 w1047]
          tunnel: w1023 -> [w1031 _]
          tunnel: w1019 -> [w1039 _]
          tunnel: w1026 -> [w1037 _]
          tunnel: w1021 -> [w1040 _]
          tunnel: w1022 -> [_ w1044]
          frame False {
            n399 = Unbundle By Name(w1031) -> ("user event"=w1038:refnum<user-event>)
            n400 = call "ClearSubPanel.vi"("error in"=w1033, "user event ref"=w1038, "sub panel ref in"=w1039) -> ("error out"=w1032:errorcluster)  [unwired: 7 in, 1 out]
            n401 = call "LoadNodeUIStandardEvents.vi"("Standard Event"=w1031, "error in"=w1032, "sub panel ref"=w1039, "main queue"=w1037, "node"=w1041) -> ("error out"=w1036:errorcluster)  [unwired: 6 in]
            n402 = property class="Pnl"(reference=w1040, error in=w1036, "DeferPanUpdts"=FALSE ("Defer Panel Updates")) -> (error out=w1035:errorcluster)  [unwired: 1 out]
          }
          frame True {
            n403 = Format Into String(format string="%s node is invalid" ("initial string"), w1044) -> (resulting string=w1042:string)  [unwired: 2 in, 1 out]
            n404 = call "CEF_error generator.vi"("error in"=w1047, "source"="TSS::ActivateNode", "append error message"=w1042, "error code (0)"=42) -> ("error out"=w1046:errorcluster)  [unwired: 5 in]
          }
        }
      }
      frame "Move" {
        n405 = Unflatten From String(type=T9 {"node ref"=refnum, "new parent"=refnum, "Index"=0} ("Cluster"), binary string=w1067, error in (no error)=w1064) -> (value=w1065:T9, error out=w1060:errorcluster)  [unwired: 2 in, 1 out]
        n406 = Unbundle By Name(w1065) -> ("Index"=w1049:i32, "node ref"=w1056:T2, "new parent"=w1068:T2)
        n407 = call "MoveNode.vi"("error in"=w1060, "index"=w1049, "new parent"=w1068, "node"=w1056) -> ("error out"=w1058:errorcluster)  [unwired: 7 in]
        n408 = call "Summary.vi"("error in"=w1058, "node self ref"=w1056) -> ("error out"=w1057:errorcluster, "summary"=w1054:T22)  [unwired: 8 in]
        n409 = Index Array(array=w1054, index=w1049) -> (element=w1055:T23)
        n410 = Unbundle By Name(w1055) -> ("ID"=w1052:string)
        n411 = Bundle By Name(cluster=w1061, "unsaved changes"=TRUE) -> (w1062:T1)
        n412 = Bundle("PopulateTree", "ID"=w1052) -> (w1050:cluster{string, "ID":string})  [unwired: 1 in]
        n413 = Enqueue Element(queue=w1051, element=w1050, error in (no error)=w1057) -> (error out=w1059:errorcluster)  [unwired: 1 in, 2 out]
      }
      frame "NodeDataChange" {
        n414 = Unbundle By Name(w1084) -> ("root"=w1071:T2)
        n415 = property class="NISE_CEF_Node"(reference=w1071) -> ("DataAccess:Children"=w1072:refnum<data-value>[])  [unwired: 1 in, 2 out]
        n416 = Index Array(array=w1072) -> (element=w1070:refnum<data-value>)  [unwired: 1 in]
        n417 = call "Find Engine from Child.vi"("error in (no error)"=w1082, "Node ID"=w1083, "HW Engine"=w1070) -> ("error out"=w1076:errorcluster, "Engine"=w1081:refnum<data-value>)  [unwired: 7 in]
        n418 = in-place {
          in-place-border: w1073 -> [w1093]
          in-place-border: w1077 -> [w1090]
          in-place-border: w1076 -> [w1092]
          in-place-border: [w1091] -> w1075
          in-place-border: [w1090] -> w1074
          in-place-border: w1069 -> [w1088]
          n419 = in-place-dvr #6(w1081) -> (w1094:refnum<class "CEF_Node.lvclass">)  [unwired: 1 out]
          n420 = call-dynamic "MenuHandler.vi"("tree control"=w1093, "main queue"=w1090, "error in"=w1092, "parameters"=w1088, "menu string"="Reset Engine" ("message value"), "CEF_Node in"=w1094) -> ("error out"=w1091:errorcluster, "CEF_Node out"=w1095:refnum<class "CEF_Node.lvclass">)  [unwired: 2 in, 2 out]
          n421 = in-place-dvr #6(w1095) -> ()  [unwired: 2 out]
        }
        n422 = Bundle By Name(cluster=w1084, "unsaved changes"=TRUE) -> (w1087:T1)
        n423 = Bundle("message name"="RefreshNode", "") -> (w1078:cluster{"message name":string, string})  [unwired: 1 in]
        n424 = Enqueue Element(queue=w1074, element=w1078, error in (no error)=w1075) -> (error out=w1085:errorcluster)  [unwired: 1 in, 2 out]
      }
      frame "-------Engine Operations-----------" {
      }
      frame "Export Engine" {
        n425 = Unbundle By Name(w1101) -> ("repository"=w1103:refnum<class "CEF_Repository.lvclass">, "current path"=w1098:path)
        n426 = call "IDtoNode.vi"("error in"=w1108, "ID"=w1107) -> ("error out"=w1104:errorcluster, "invalid Id"=w1106:bool, "node ref"=w1105:refnum<data-value>)  [unwired: 7 in]
        n427 = case shown="False" w1106 {
          tunnel: w1105 -> [w1113 _]
          tunnel: w1104 -> [w1110 w1135]
          tunnel: w1103 -> [w1118 w1132]
          tunnel: [w1116 w1134] -> w1102
          tunnel: [w1115 w1132] -> w1099
          tunnel: w1098 -> [w1114 _]
          frame False {
            n428 = property class="NISE_CEF_Node"(reference=w1113, error in=w1110) -> (reference out=w1111:refnum<data-value>, error out=w1109:errorcluster, "DataAccess:NodeClass"=w1112:string)
            n429 = call "FileDialog.vi"("error in"=w1109, "default name"=w1112, "start path"=w1114) -> ("error out"=w1119:errorcluster, "cancelled"=w1120:bool, "selected path"=w1117:path)  [unwired: 6 in]
            n430 = case shown="False" w1120 {
              tunnel: w1119 -> [w1128 w1129]
              tunnel: w1111 -> [w1127 _]
              tunnel: w1118 -> [w1126 w1130]
              tunnel: w1117 -> [w1121 _]
              tunnel: [w1123 w1129] -> w1116
              tunnel: [w1122 w1130] -> w1115
              frame False {
                n431 = call-dynamic "ReadTree.vi"("error in"=w1128, "root"=w1127, "CEF_Repository in"=w1126) -> ("error out"=w1124:errorcluster, "CEF_Repository out"=w1125:refnum<class "CEF_Repository.lvclass">)  [unwired: 7 in]
                n432 = call-dynamic "Save.vi"("error in"=w1124, "file path"=w1121, "CEF_Repository in"=w1125) -> ("error out"=w1123:errorcluster, "CEF_Repository out"=w1122:refnum<class "CEF_Repository.lvclass">)  [unwired: 7 in]
              }
              frame True {
              }
            }
          }
          frame True {
            n433 = call "CEF_error generator.vi"("error in"=w1135, "source"="TSS::Export Engine", "append error message"="Invalid Node" ("source"), "error code (0)"=42) -> ("error out"=w1134:errorcluster)  [unwired: 5 in]
          }
        }
        n434 = Bundle By Name(cluster=w1101, "repository"=w1099) -> (w1100:T1)
      }
      frame "Import Engine" {
        n435 = Unbundle By Name(w1148) -> ("root"=w1139:T2, "repository"=w1151:refnum<class "CEF_Repository.lvclass">, "current path"=w1144:path)
        n436 = call "IDtoNode.vi"("error in"=w1143, "ID"=w1138) -> ("error out"=w1142:errorcluster, "node ref"=w1141:refnum<data-value>)  [unwired: 7 in, 1 out]
        n437 = call "FileDialog.vi"("error in"=w1142, "start path"=w1144) -> ("error out"=w1152:errorcluster, "cancelled"=w1145:bool, "selected path"=w1149:path)  [unwired: 7 in]
        n438 = case shown="False" w1145 {
          tunnel: w1152 -> [w1163 w1195]
          tunnel: w1151 -> [w1162 w1194]
          tunnel: w1150 -> [w1159 _]
          tunnel: w1149 -> [w1155 _]
          tunnel: [w1158 w1193] -> w1140
          tunnel: [w1157 w1194] -> w1137
          tunnel: [w1156 w1195] -> w1146
          tunnel: w1141 -> [w1154 _]
          tunnel: w1139 -> [w1153 w1193]
          frame False {
            n439 = call-dynamic "Open.vi"("error in"=w1163, "file path"=w1155, "CEF_Repository in"=w1162) -> ("error out"=w1160:errorcluster, "invalid?"=w1164:bool, "CEF_Repository out"=w1161:refnum<class "CEF_Repository.lvclass">)  [unwired: 6 in]
            n440 = case shown="False" w1164 {
              tunnel: [w1182 w1183] -> w1157
              tunnel: [w1179 w1191] -> w1156
              tunnel: [w1170 w1186] -> w1158
              tunnel: w1161 -> [w1180 w1183]
              tunnel: w1160 -> [w1181 w1192]
              tunnel: w1159 -> [w1165 _]
              tunnel: w1155 -> [_ w1188]
              tunnel: w1154 -> [w1178 _]
              tunnel: w1153 -> [w1175 w1186]
              frame False {
                n441 = call-dynamic "WriteTree.vi"("error in"=w1181, "CEF_Repository in"=w1180) -> ("error out"=w1176:errorcluster, "root"=w1177:refnum<data-value>, "CEF_Repository out"=w1182:refnum<class "CEF_Repository.lvclass">)  [unwired: 7 in]
                n442 = call "LinkNodes.vi"("error in"=w1176, "child in"=w1177, "parent in"=w1178) -> ("error out"=w1174:errorcluster, "parent out"=w1172:refnum<data-value>)  [unwired: 6 in, 1 out]
                n443 = call "LinkNodes.vi"("error in"=w1174, "child in"=w1172, "parent in"=w1175) -> ("error out"=w1173:errorcluster, "parent out"=w1171:refnum<data-value>)  [unwired: 6 in, 1 out]
                n444 = Bundle("PopulateTree", "") -> (w1166:cluster{string, string})  [unwired: 1 in]
                n445 = call "UnlinkNode.vi"("error in"=w1173, "child in"=w1172, "parent in"=w1171) -> ("error out"=w1169:errorcluster, "parent out"=w1170:refnum<data-value>)  [unwired: 6 in, 1 out]
                n446 = Enqueue Element(queue=w1165, element=w1166, error in (no error)=w1169) -> (error out=w1179:errorcluster)  [unwired: 1 in, 2 out]
              }
              frame True {
                n447 = Strip Path(path=w1188) -> (name=w1187:string)  [unwired: 1 out]
                n448 = Format Into String(format string="%s config invalid " ("source"), w1187) -> (resulting string=w1185:string)  [unwired: 2 in, 1 out]
                n449 = call "CEF_error generator.vi"("error in"=w1192, "source"="TSS::Import Engine", "append error message"=w1185, "error code (0)"=42) -> ("error out"=w1191:errorcluster)  [unwired: 5 in]
              }
            }
          }
          frame True {
          }
        }
        n450 = Bundle By Name(cluster=w1148, "repository"=w1137, "root"=w1140) -> (w1147:T1)
      }
      frame "Control Engines" {
        # "Engines"
        # "0 : HW Engine\n1 : Special Test"
        n451 = Unbundle By Name(w1214) -> ("root"=w1215:T2)
        n452 = Unflatten From String(type=TRUE, binary string=w1207, error in (no error)=w1208) -> (value=w1205:bool, error out=w1201:errorcluster)  [unwired: 2 in, 1 out]
        n453 = property class="NISE_CEF_Node"(reference=w1215) -> ("DataAccess:Children"=w1213:refnum<data-value>[])  [unwired: 1 in, 2 out]
        n454 = Index Array(array=w1213) -> (element=w1212:refnum<data-value>)  [unwired: 1 in]
        n455 = Bundle("PopulateTree", "") -> (w1204:cluster{string, string})  [unwired: 1 in]
        n456 = property class="NISE_CEF_Node"(reference=w1212) -> ("DataAccess:Children"=w1211:refnum<data-value>[])  [unwired: 1 in, 2 out]
        n457 = Enqueue Element(queue=w1199, element=w1204, error in (no error)=w1201) -> (error out=w1200:errorcluster)  [unwired: 1 in, 2 out]
        n458 = for {
          tunnel: w1211 -> [w1222] mode=indexing
          shift-right: [w1225] -> w1198
          shift-left: w1200 -> [w1221]
          tunnel: w1210 -> [w1223]
          tunnel: w1209 -> [w1220]
          tunnel: w1199 -> [w1224]
          tunnel: w1205 -> [w1219]
          n459 = in-place {
            in-place-border: w1221 -> [w1226]
            in-place-border: [w1231] -> w1225
            in-place-border: w1224 -> [w1229]
            in-place-border: w1223 -> [w1233]
            in-place-border: w1220 -> [w1230]
            in-place-border: w1219 -> [w1227]
            n460 = in-place-dvr #7(w1222) -> (w1234:refnum<class "CEF_Node.lvclass">)  [unwired: 1 out]
            n461 = case shown="True" w1227 {
              tunnel: ["Reset Engine" ("message value") "Initialize Engine" ("message value")] -> w1228
              frame False {
              }
              frame True {
                n462 = Wait (ms)(milliseconds to wait=u32 300) -> ()  [unwired: 1 out]
              }
            }
            n463 = call-dynamic "MenuHandler.vi"("tree control"=w1233, "main queue"=w1229, "error in"=w1226, "parameters"=w1230, "menu string"=w1228, "CEF_Node in"=w1234) -> ("error out"=w1231:errorcluster, "CEF_Node out"=w1232:refnum<class "CEF_Node.lvclass">)  [unwired: 2 in, 2 out]
            n464 = in-place-dvr #7(w1232) -> ()  [unwired: 2 out]
          }
        }
        n465 = case shown="False" w1197 {
          tunnel: w1198 -> [w1217 w1218]
          tunnel: [w1216 w1218] -> w1196
          frame False {
            n466 = invoke class="VI" method="FP.Open"(error in=w1217) -> (error out=w1216:errorcluster)  [unwired: 4 in, 4 out]
          }
          frame True {
          }
        }
      }
      frame "Record Engines" {
        n467 = Unflatten From String(type=TRUE, binary string=w1245, error in (no error)=w1246) -> (value=w1244:bool, error out=w1243:errorcluster)  [unwired: 2 in, 1 out]
        n468 = case shown="False" w1244 {
          selector: w1244 -> [_ w1267]
          tunnel: w1243 -> [w1254 w1259]
          tunnel: [w1250 w1265] -> w1242
          tunnel: w1241 -> [w1253 w1269]
          tunnel: [w1252 w1268] -> w1240
          tunnel: w1239 -> [_ _]
          tunnel: w1238 -> [_ _]
          frame False {
            n469 = Unbundle By Name(w1253) -> ("tdms file"=w1249:refnum<k34>)
            n470 = TDMS Close(8:w1254, 11:w1249) -> (0:w1250:errorcluster)  [unwired: 1 out]
            n471 = Bundle By Name(cluster=w1253, "tdms file"=refnum<k34> refnum, "Record"=FALSE) -> (w1252:T1)
          }
          frame True {
            n472 = Unbundle By Name(w1269) -> ("paths.Data"=w1262:path)
            n473 = Get Date/Time In Seconds() -> (seconds since 1Jan1904=w1263:timestamp)
            n474 = Format Into String(format string="%<%Y%m%d_%H%M%S>T.tdms", w1263) -> (resulting string=w1261:string)  [unwired: 2 in, 1 out]
            n475 = Build Path(base path=w1262, name or relative path=w1261) -> (appended path=w1260:path)
            n476 = TDMS Open(5:FALSE ("create index file? (T)"), 8:w1259, 10:T20."open or create" ("operation (0:open)"), 11:w1260) -> (0:w1258:errorcluster, 3:w1255:refnum<k34>)  [unwired: 3 in]
            n477 = case shown="No Error" w1258 {
              selector: w1258 -> [w1271 w1278]
              tunnel: [w1275 w1278] -> w1265
              tunnel: w1267 -> [_ w1280]
              tunnel: [TRUE ("Record") FALSE ("Record")] -> w1266
              frame No Error {
                n478 = property on="Time" class="DigNum (strict)"(error in=w1271, "Value"=0.0 ("Time")) -> (error out=w1270:errorcluster)  [unwired: 1 in, 1 out]
                n479 = call "Timing FGV.vi"("Time Target (s)"=5, "Timer Mode"=T19."Start Timer", "Error In"=w1270) -> ("Error Out"=w1275:errorcluster)  [unwired: 6 in, 2 out]
              }
              frame Error {
                n480 = Not(x=w1280) -> (.not. x?=w1279:bool)
                n481 = property on="Record" class="Bool (strict)"("Value"=w1279) -> ()  [unwired: 2 in, 2 out]
              }
            }
            n482 = Bundle By Name(cluster=w1269, "tdms file"=w1255, "Record"=w1266) -> (w1268:T1)
          }
        }
      }
    }
  }
  n483 = Merge Errors(w22, w24) -> (w23:errorcluster)
  n484 = Unregister For Events(event registration refnum=w17) -> ()  [unwired: 1 in, 1 out]
  n485 = call "DestroyStandardEvents.vi"("error in"=w23, "standard events"=w16) -> ()  [unwired: 9 in, 1 out]
